vi "main 0.8.vi"() -> ()   [LabVIEW 2020]
uses:
  subvi/Newport ESP301/Newport ESP301.lvlib
  subvi/sp_manip.llb/sp_manip_lib.lvlib
  subvi/sp_manip.llb/tcp_gateway.lvlib
  subvi/PHOIBOS/DEFINITIONS/DEF_dev_type.ctl
  subvi/PHOIBOS/DEFINITIONS/DEF_dev_state.ctl
  <vilib>/Utility/file.llb/Write Delimited Spreadsheet (DBL).vi
panel:
  in  "BasePath":path=path "Z:/PESdata"
  in  "cam_liveavg":bool caption="live average"
  out "G2":dbl[](graph)
  out "cam_fps":dbl=19.67681433793903 caption="FPS" format="%.1g"
  out "sideimg":dbl[][](graph)
  out "RunNumber":u16=4
  out "sum":dbl=3886353.0 format="%#.2g"
  out "max":dbl=54.0
  out "mainimg":dbl[][](graph)
  out "ESP_con?":bool=TRUE caption="ESP301"
  out "phoib_con?":bool caption="PHOIBOS"
  out "manip_con?":bool caption="manipulator"
  out "cam_con?":bool caption="camera"
  in  "main_close":bool
  in  "Tab Control":T1(tab)
  in  "manip_deltas":dbl[](array[numeric])=[0.0, 0.0, 0.0, 0.0, 0.0, 0.0] caption="delta" format="%#.5g"
  in  "aq.mode":enum32{"Radio Selection 1", "Radio Selection 2"}(radio)
  out "snap_prog":dbl(slide) scale=0.0..1.0
  in  "upper threshold":i32=1500
  in  "dark avg":i32=20
  in  "averages":i32=20 caption="N"
  in  "ESP_delta":dbl caption="relative [mm]"
  in  "ESP_-":bool
  in  "ESP_+":bool
  in  "ESP_go":bool
  in  "ESP_dest_t":dbl caption="[fs]"
  in  "ESP_dest":dbl=33.3075 caption="[mm]"
  in  "ESP_set_t0":bool
  in  "phoib_I_6s":dbl=3200.0
  in  "phoib_I_5s":dbl=1400.0
  in  "phoib_I_4s":dbl=4.2
  in  "phoib_I_3s":dbl
  in  "phoib_I_2s":dbl=35.0
  in  "phoib_I_1s":dbl=21.9
  in  "phoib_standby":bool
  in  "phoib_set":bool
  out "phoib_I_6":dbl caption="Screen Voltage"
  out "phoib_I_5":dbl caption="Detctor Voltage"
  out "phoib_I_4":dbl caption="Work Function"
  out "phoib_I_3":dbl caption="Coil Current"
  out "phoib_I_2":dbl caption="Pass Energy"
  out "phoib_I_1":dbl caption="Kinetic Energy"
  out "Saved Positions":string[][](table)=[["ertwertwert", "-2.299945", "-2.030214", "38.900024", "50.000762", "0.000887", "-97.998082"], ["uztgugt", "-14.999451", "-13.638894", "442.380066", "13.998380", "-1.893758", "-76.305838"], ["asdf", "-14.999451", "-13.638894", "442.380066", "13.998380", "-1.893758", "-76.305838"], ["test3", "-14.999451", "-13.638894", "441.380066", "13.998380", "-1.893758", "-76.305838"]]
  in  "Save Pos":bool
  in  "Load":bool
  in  "Delete":bool
  in  "ManipRel +":bool
  in  "ManipRel -":bool
  in  "Move Abs":bool
  in  "stop manip":bool
  in  "dest":dbl[](array[numeric])=[0.007141549166819264, -0.009888298846365134, 431.30615234375, 89.00040512814502, 1.109125024699864, -227.9162918846475] caption="destination" format="%#.5g"
  out "axis":string[](array[string])=["x", "y", "z", "polar", "tilt", "azimut"]
  out "pos":dbl[](array[numeric])=[0.007141549166819264, -0.009888298846365134, 431.30615234375, 89.00040512814502, 1.109125024699864, -227.9162918846475] caption="position" format="%.5f"
  in  "Mode":T2(ring)=enum."WideAngleMode"
  in  "VoltageRange":enum16{"3.5kV", "1.5kV", "400V", "100V", "10V"}(ring)=enum."400V"
  out "ESP_pos":dbl=33.3075 caption="Position"
  out "ESP_delay":dbl caption="Delay"
  out "ESP_t0":dbl=33.3075 caption="Time Zero @"
  out "phoib_I_7":dbl caption="Conversion Voltage"
  in  "phoib_I_7s":dbl
  in  "phoib_I_8s":dbl
  in  "phoib_I_9s":dbl
  out "phoib_I_8":dbl caption="FD1"
  out "phoib_I_9":dbl caption="FD2"
  in  "gain":bool
  in  "exposure [ms]":u32=20
  in  "binning":u16(ring)=2 items=["X 1", "X 2", "X 4", "X 8"]
  in  "cam_dark?":bool caption="subtract dark?"
  in  "cam_dark":bool
  in  "cam_saveimg":bool
  in  "e-size":u8
  in  "lower threshold":i32=100
  in  "count?":bool
  out "ETA":timestamp format="%<%H:%M:%S>T"
  in  "ROI Left":i32=1
  in  "ROI Right":i32=40
  in  "ROI Top":i32=1
  in  "ROI Bottom":i32=32
  in  "delscan_iters":u32 caption="iterations"
  out "scangraph":cluster{dbl[], dbl[]}(graph)
  in  "delscan_abort":bool
  out "delscan_progress":u32(slide) scale=0.0..20.0
  in  "delscan_go":bool
  out "delscan_pos":dbl caption="current delay [fs]"
  in  "delscan_end":dbl caption="end [fs]"
  in  "delscan_stepsize":dbl caption="stepsize [fs]"
  in  "delscan_start":dbl caption="start [fs]"
  in  "comment":string
  out "iteration":i32
  out "opti_frames":dbl=25.0 caption="#steps_opti"
  out "opti_current_frame":i32=25
  out "Measurement Progress":u8(slide) scale=0.0..100.0
  out "Camera Aquisition":u8(slide) scale=0.0..100.0
  in  "Optimize":bool
  in  "OptiStepSize":dbl=-1.0 caption="Step Size"
  in  "OptiRange":dbl=25.0 caption="Range"
  in  "meas_axis":string(combo)="tilt" caption="Axis"
  in  "meas_avg":i32=60 caption="Frames2Average"
  in  "OptiCancel":bool
  out "#steps_opti":dbl=25.0
  out "current_step_opti":i32=25
  out "ETA":string
  out "manip_error":errorcluster
  out "esp_error":errorcluster
  in  "manip_init":bool
  in  "manip_release":bool
  in  "phoib_init":bool
  in  "phoib_release":bool
  in  "ESP_init":bool
  in  "ESP_release":bool
  in  "ESP301 VISA":refnum<visa-resource-name>="COM8"
  in  "board number":i32
  in  "cam_init":bool
  in  "cam_release":bool
  out "cam_error":errorcluster
  out "phoib_error":errorcluster
  out "state":T3 items=["Off"=-1, "Standby"=0, "On"=1]
  in  "ESP Axis":i32=1 min=1 max=3
  # "camera"
  # "analyzer"
  # "manipulator"
  # "aquisition"
  # "delay stage"
  # "Position"
  # "Destination"
  # "step _ of _"
  # "step _ of _"
  # "camera"
  # "phoibos"
  # "ESP301"
  # "manipulator"
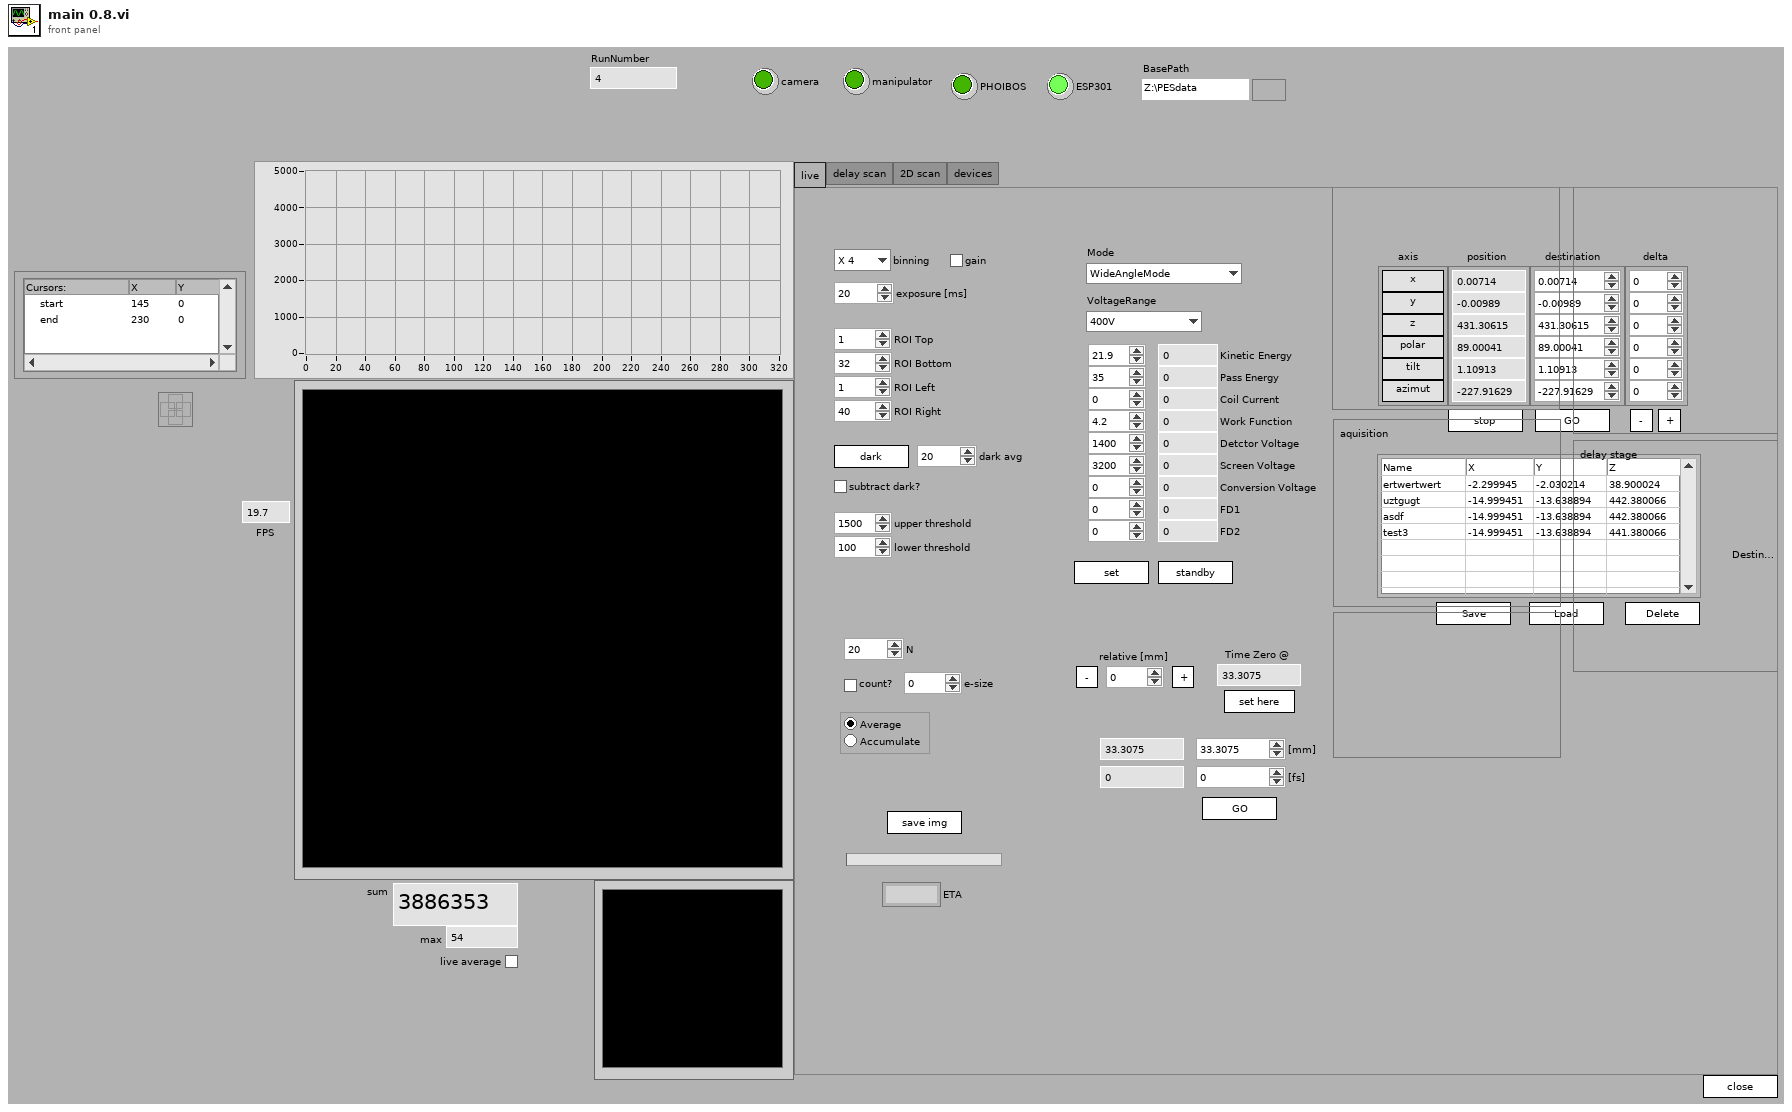
[diagram p1: front panel]
types:
  T1 = enum32{"live", "delay scan", "2D scan", "devices"}
  T2 = enum16{"HighMagnification", "MediumMagnification", "LowMagnification", "HighAngularDispersion", "MediumAngularDispersion", "LowAngularDispersion", "WideAngleMode", "LargeArea", "MediumArea", "SmallArea", "HighMagnification2", "SmallArea2", "ImagingMode"}
  T3 = typedef "DEF_dev_state.ctl" = i32
  T4 = typedef "LVCursorListTypeDef.ctl" = cluster{"Name":string, "Color":u32, "Style":u8, "Point Style":u8, "Name Visible":bool, "Allow Drag":bool, "Cursor Mode":u32, "Plot":i32, "Index":i32, "Position":cluster{"X":dbl, "Y":dbl}, "X Scale":u32, "Y Scale":u32, "Watch Plots":i32[], "Watch All Plots":bool, "Plot Area":i32, "Label Offset":cluster{"X":dbl, "Y":dbl}}[]
  T5 = cluster{"Name":string, "Color":u32, "Style":u8, "Point Style":u8, "Name Visible":bool, "Allow Drag":bool, "Cursor Mode":u32, "Plot":i32, "Index":i32, "Position":cluster{"X":dbl, "Y":dbl}, "X Scale":u32, "Y Scale":u32, "Watch Plots":i32[], "Watch All Plots":bool, "Plot Area":i32, "Label Offset":cluster{"X":dbl, "Y":dbl}}
  T6 = cluster{"Camera type":u32, "Operating mode\nHP & QE / HS & DiCam Pro ":u32, "Frame trigger \n(High Performance and QE only)":u16, "Sequence trigger":u16, "Low Light\n(QE only)":bool, "Gain":bool, "Horzontal\nbinning":u16, "Vertical\nbinning ":u16, "ROI Left":i32, "ROI Right":i32, "ROI Top":i32, "ROI Bottom":i32}
  T7 = cluster{"Axis_Name":string, "Axis_Type":string, "Axis_Position":dbl, "continous":bool, "moving":bool}[]
  T8 = typedef "DEF_dev_type.ctl" = enum32{"devA (analyzer)", "devD (detector)"}
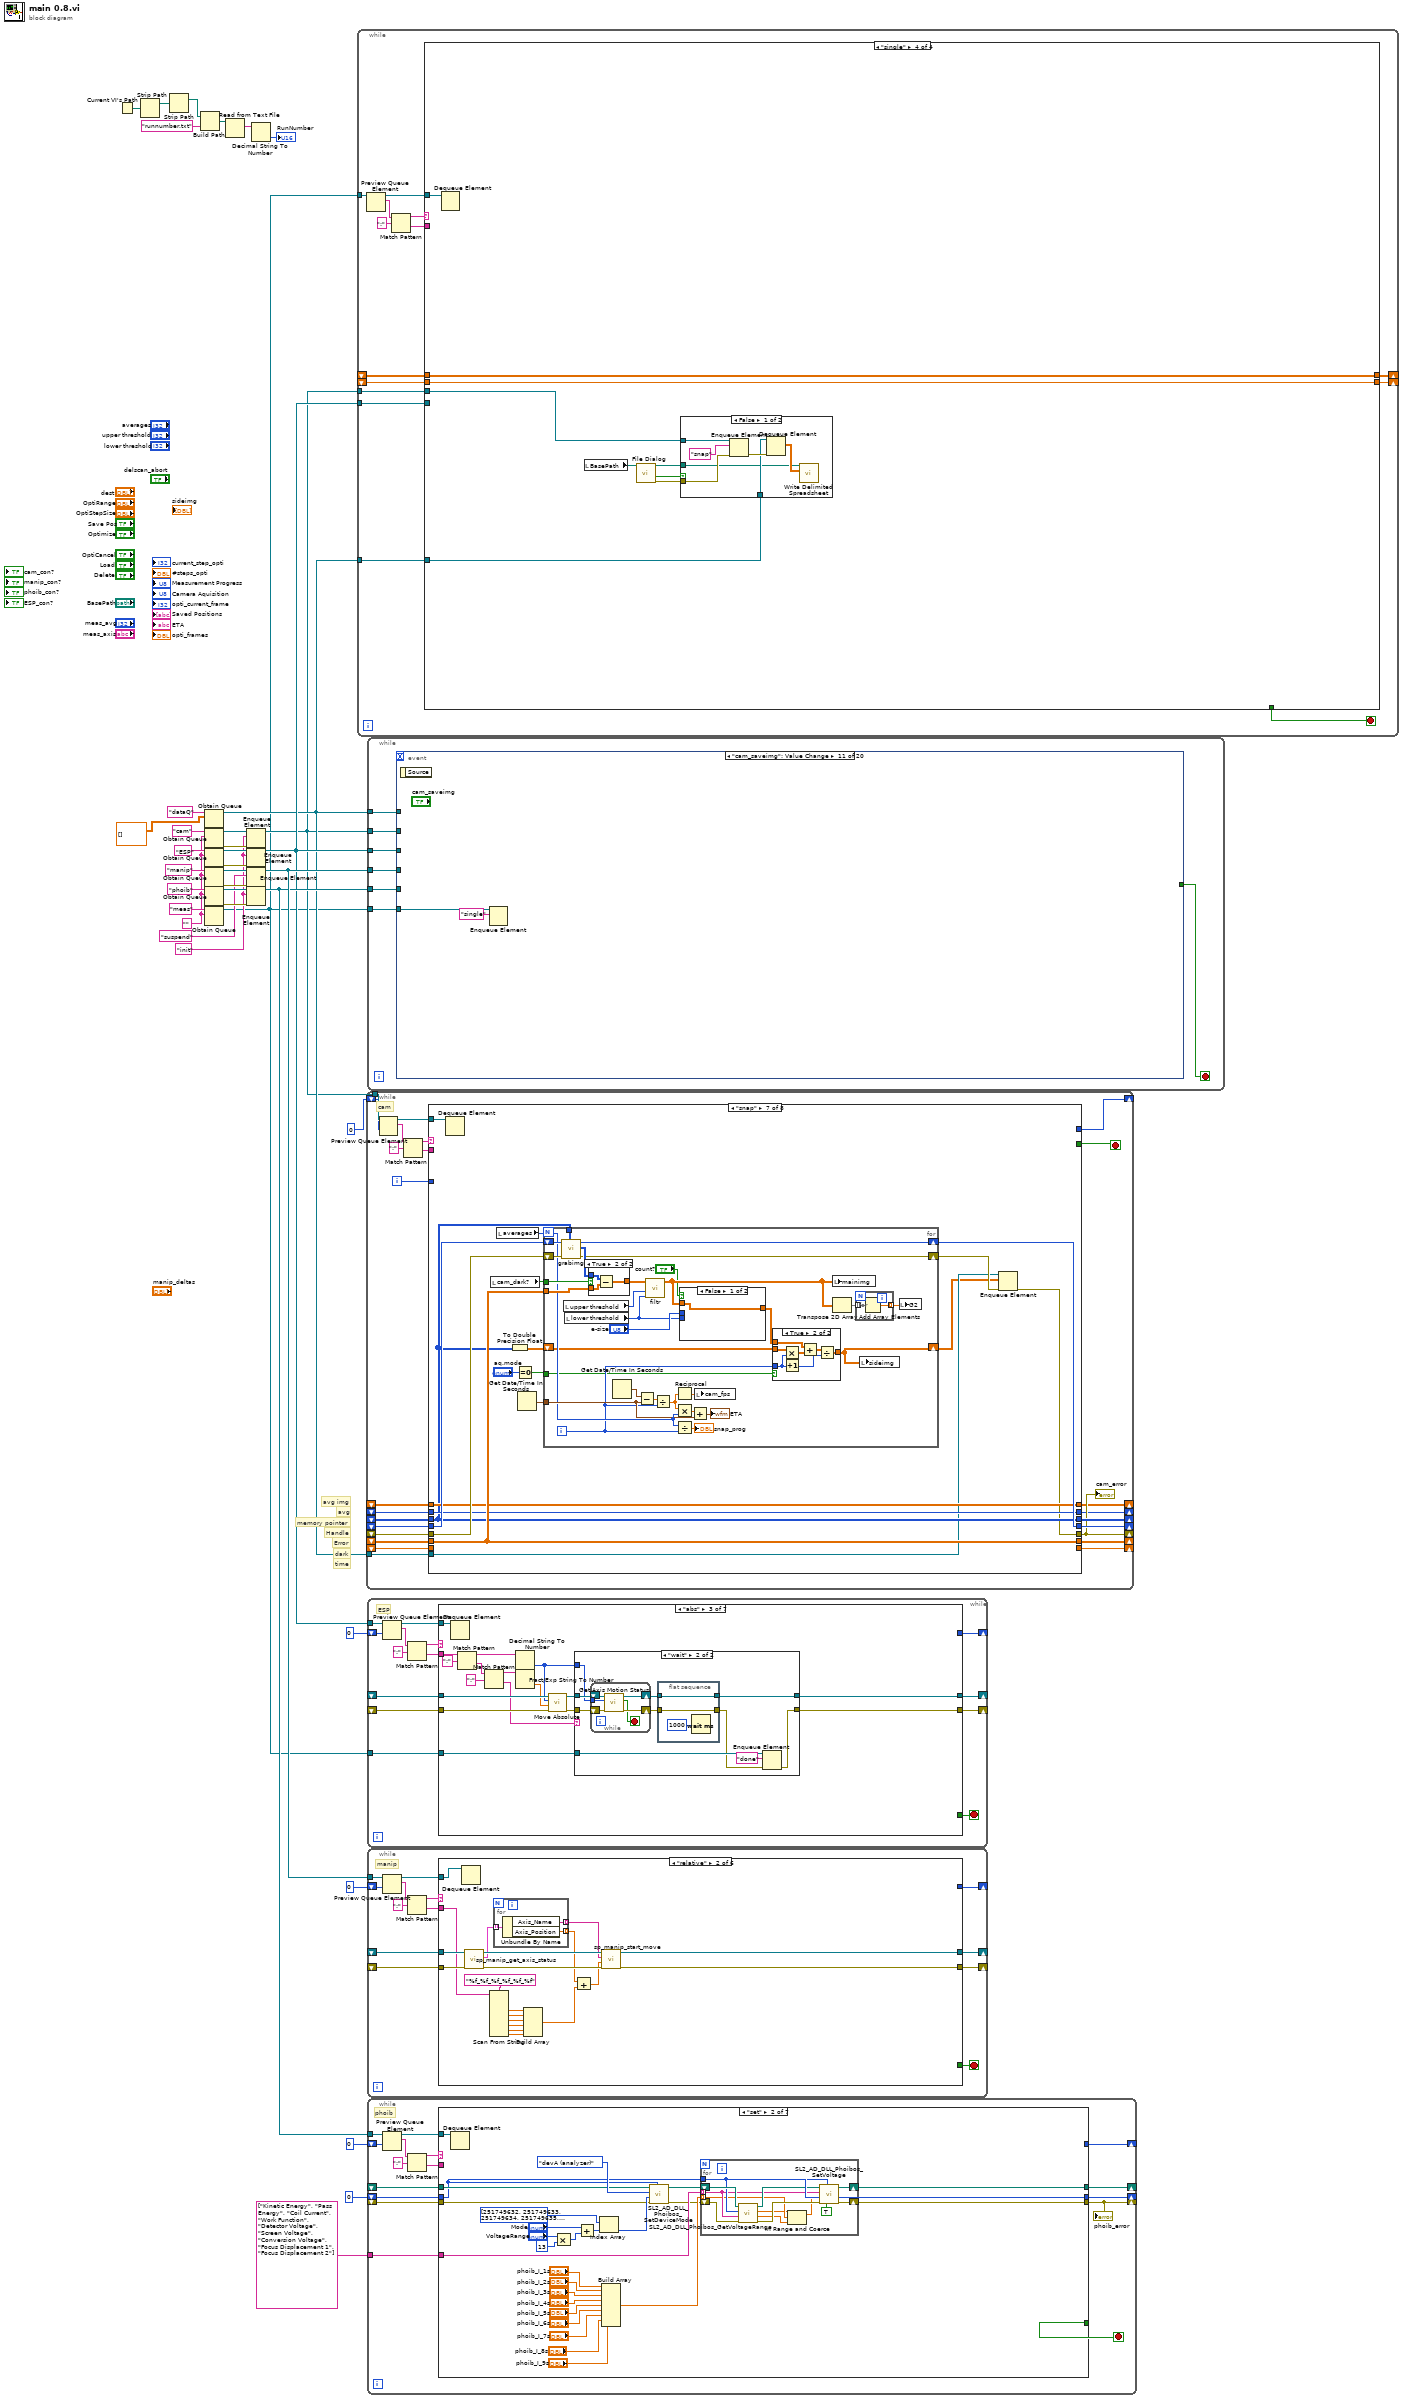
[diagram p0: block diagram]
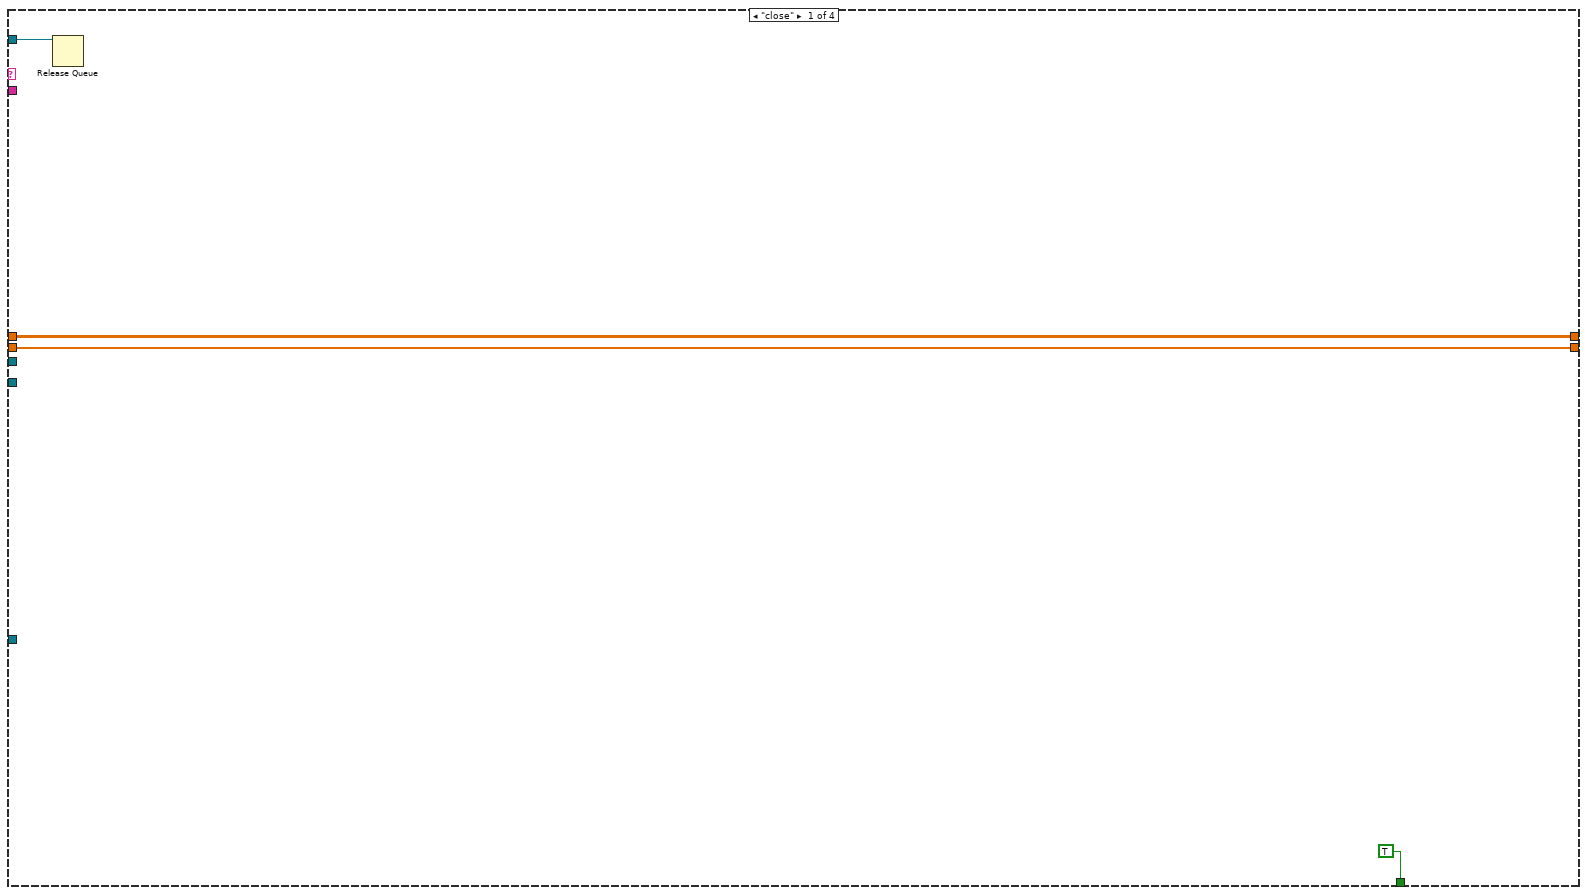
[diagram p2: hidden frame]
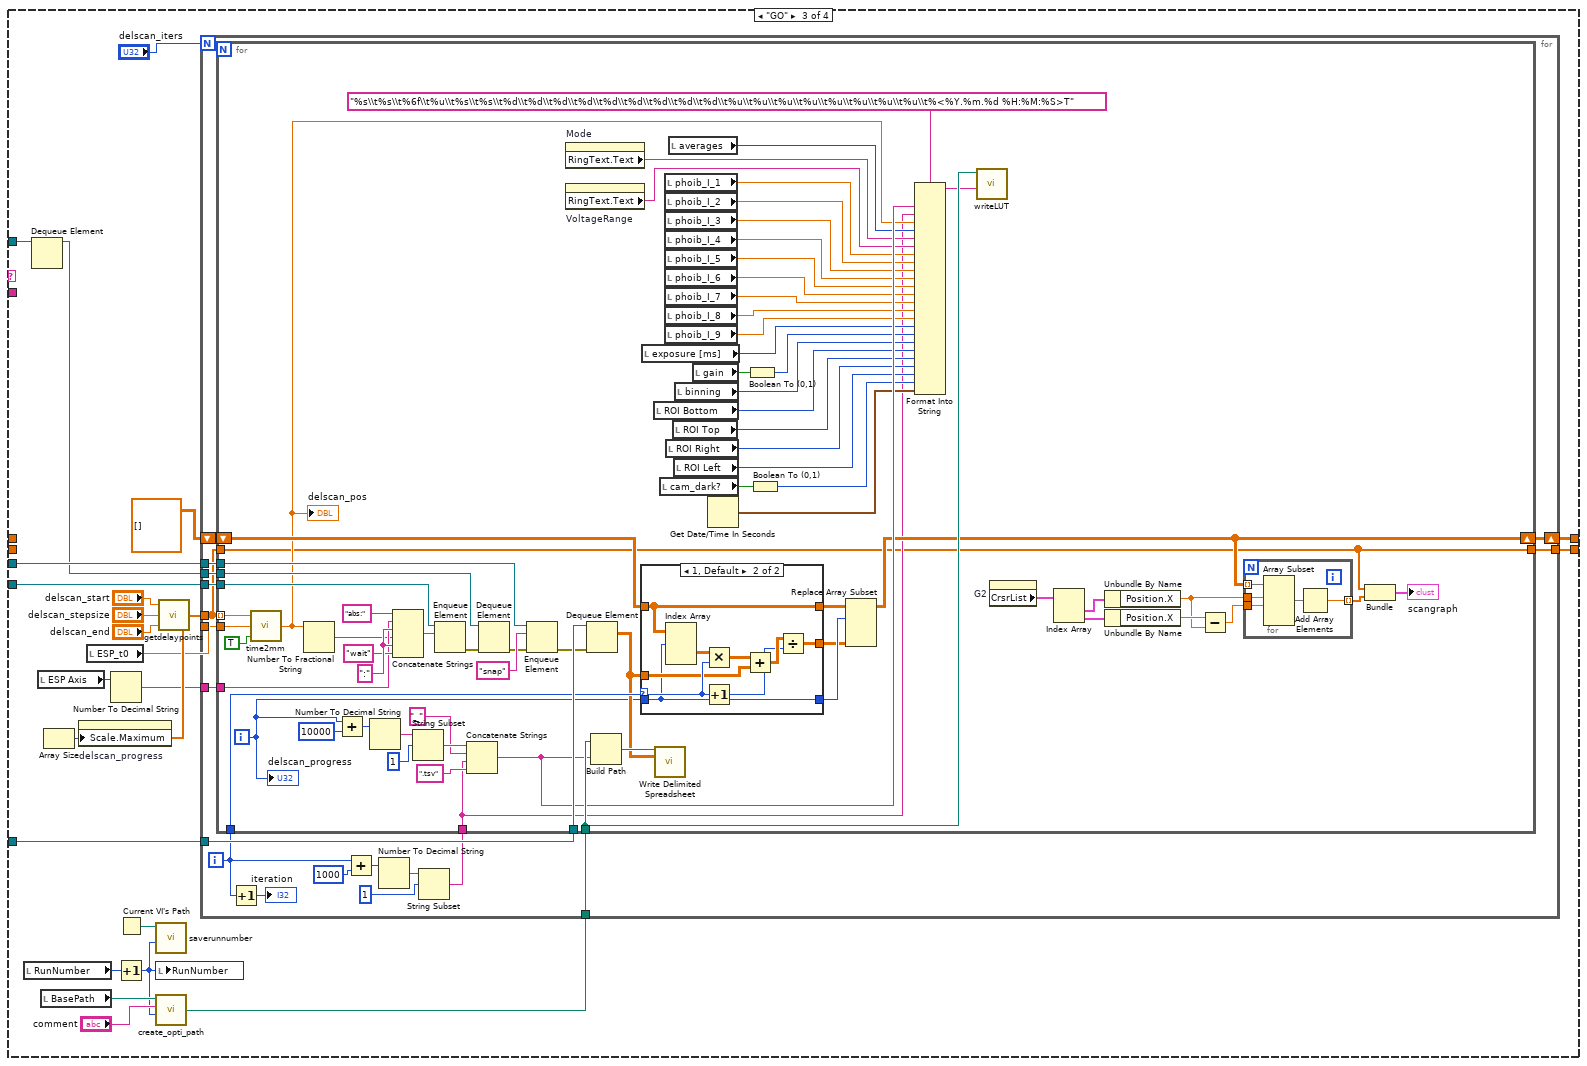
[diagram p4: hidden frame]
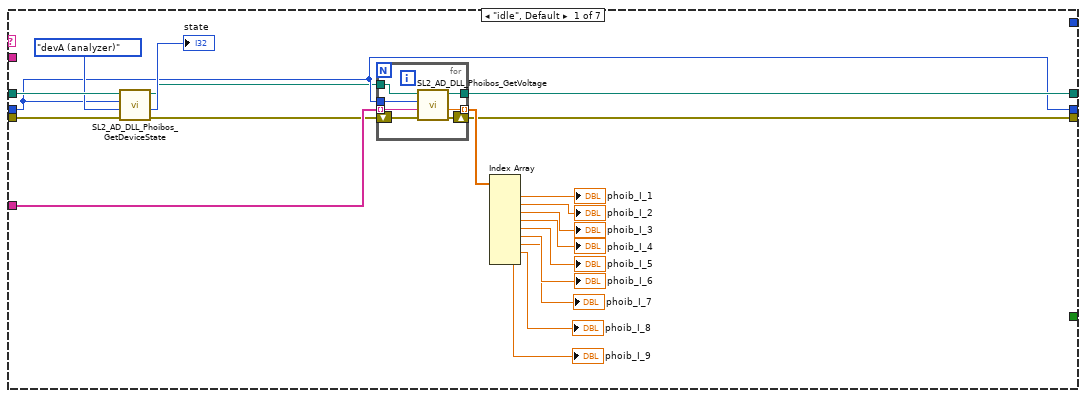
[diagram p7: hidden frame]
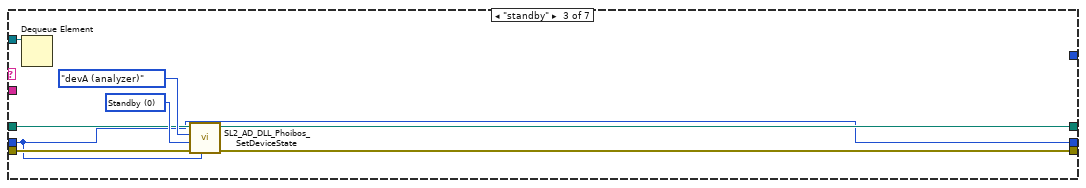
[diagram p8: hidden frame]
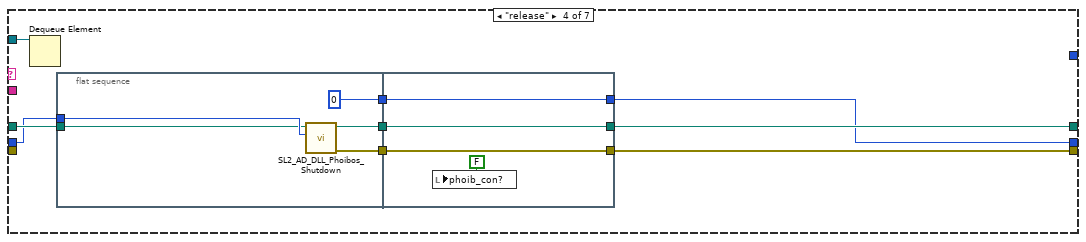
[diagram p9: hidden frame]
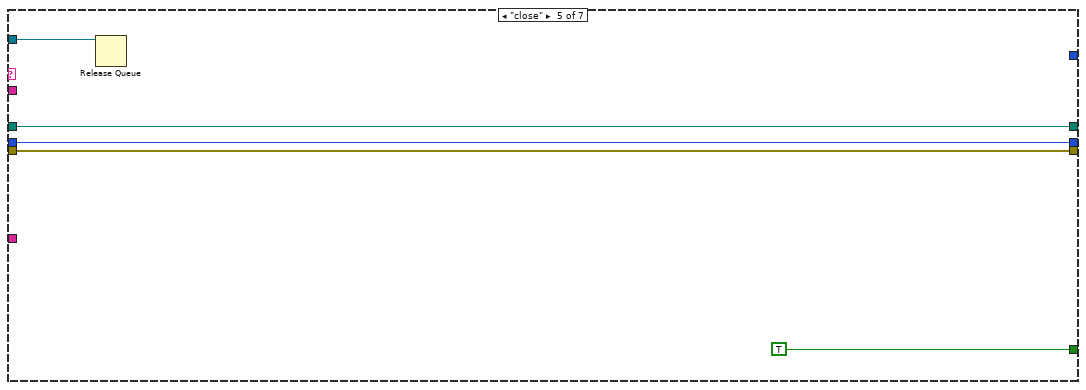
[diagram p10: hidden frame]
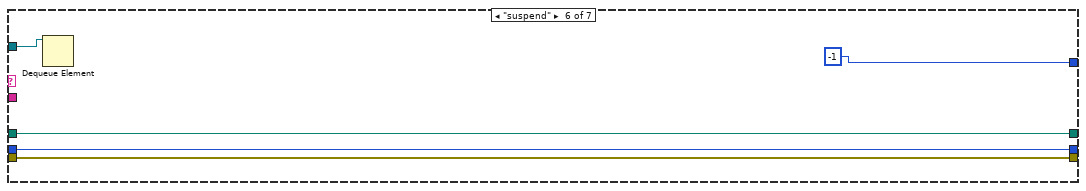
[diagram p11: hidden frame]
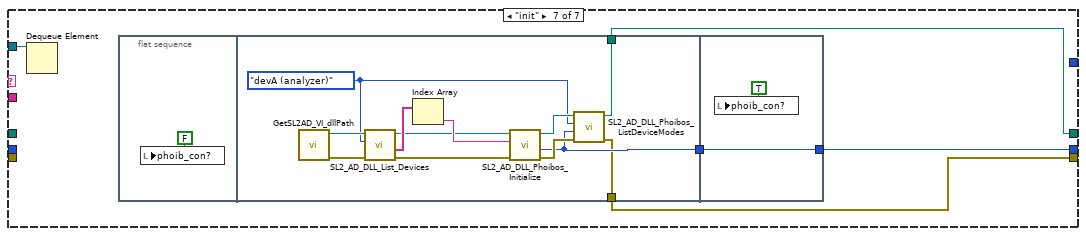
[diagram p12: hidden frame]
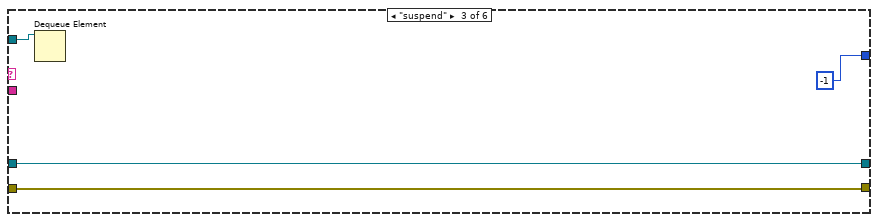
[diagram p14: hidden frame]
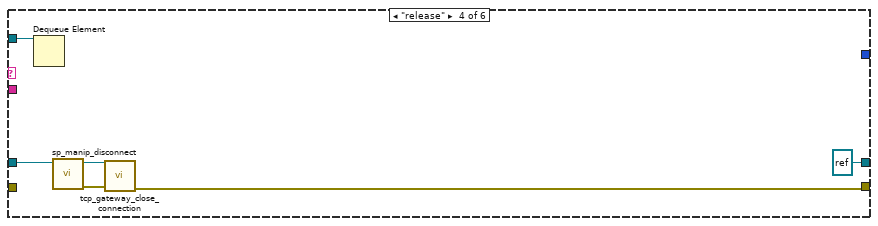
[diagram p15: hidden frame]
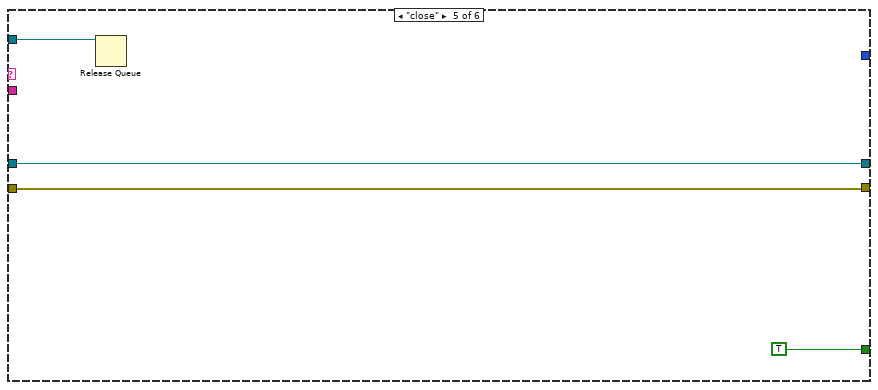
[diagram p16: hidden frame]
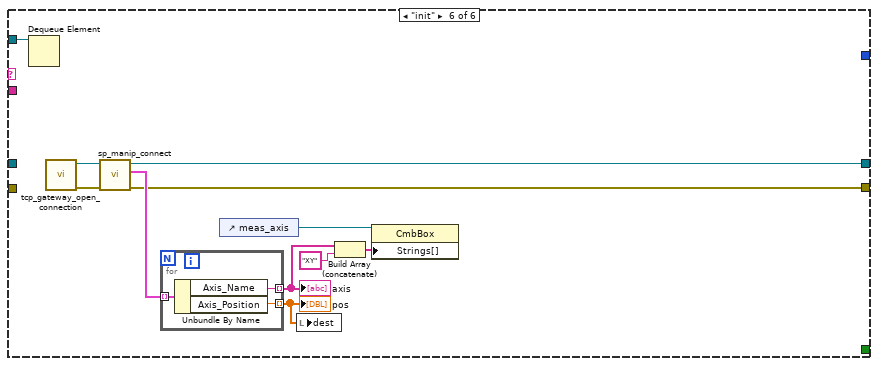
[diagram p17: hidden frame]
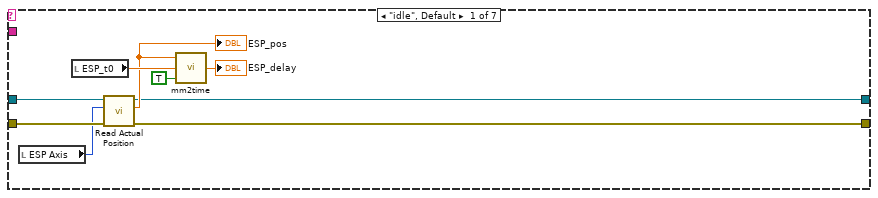
[diagram p18: hidden frame]
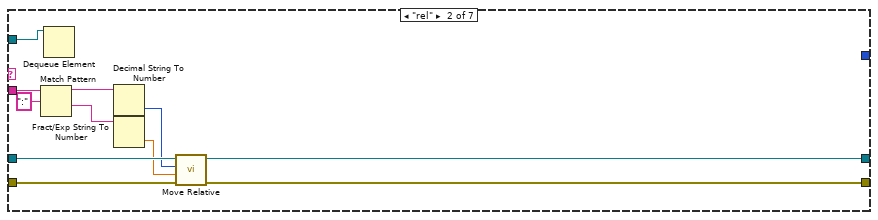
[diagram p19: hidden frame]
diagram:
  w13 = "init" ("name (unnamed)")
  w15 = "" ("name (unnamed)")
  # "avg img"
  # "avg"
  # "time"
  # "dark"
  # "Error"
  # "Handle"
  # "memory pointer"
  n1 = Current VI's Path() -> (path=w2:path)
  n2 = Strip Path(path=w2) -> (stripped path=w7:path)  [unwired: 1 out]
  n3 = Strip Path(path=w7) -> (stripped path=w8:path)  [unwired: 1 out]
  n4 = Build Path(base path=w8, name or relative path="runnumber.txt") -> (appended path=w4:path)
  n5 = Obtain Queue(name (unnamed)="dataQ", element data type=dbl[][] []) -> (queue out=w10:refnum<queue>)  [unwired: 3 in, 2 out]
  n6 = Obtain Queue(name (unnamed)="cam", element data type=w15) -> (queue out=w36:refnum<queue>, error out=w35:errorcluster)  [unwired: 3 in, 1 out]
  n7 = Obtain Queue(name (unnamed)="ESP", element data type=w15) -> (queue out=w33:refnum<queue>, error out=w34:errorcluster)  [unwired: 3 in, 1 out]
  n8 = Obtain Queue(name (unnamed)="manip", element data type=w15) -> (queue out=w30:refnum<queue>, error out=w29:errorcluster)  [unwired: 3 in, 1 out]
  n9 = Obtain Queue(name (unnamed)="phoib", element data type=w15) -> (queue out=w27:refnum<queue>, error out=w28:errorcluster)  [unwired: 3 in, 1 out]
  n10 = Obtain Queue(name (unnamed)="meas", element data type=w15) -> (queue out=w1:refnum<queue>)  [unwired: 3 in, 2 out]
  n11 = Read from Text File(file (use dialog)=w4) -> (text=w5:string)  [unwired: 3 in, 3 out]
  n12 = Enqueue Element(queue=w36, element=w13, error in (no error)=w35) -> (queue out=w9:refnum<queue>)  [unwired: 1 in, 2 out]
  n13 = Enqueue Element(queue=w33, element=w13, error in (no error)=w34) -> (queue out=w12:refnum<queue>)  [unwired: 1 in, 2 out]
  n14 = Enqueue Element(queue=w30, element="suspend" ("name (unnamed)"), error in (no error)=w29) -> (queue out=w24:refnum<queue>)  [unwired: 1 in, 2 out]
  n15 = Enqueue Element(queue=w27, element=w13, error in (no error)=w28) -> (queue out=w23:refnum<queue>)  [unwired: 1 in, 2 out]
  n16 = Decimal String To Number(string=w5) -> (number=→"RunNumber":i32)  [unwired: 2 in, 1 out]
  n17 = while {
    tunnel: w10 -> [w51]
    tunnel: w12 -> [w50]
    tunnel: w9 -> [w49]
    shift-right: [w46] -> _
    shift-left: _ -> [w48]
    shift-right: [w45] -> _
    shift-left: _ -> [w47]
    tunnel: w1 -> [w42]
    stop <- w38 stop-if-true
    n18 = Preview Queue Element(queue=w42) -> (queue out=w39:refnum<queue>, element=w44:string)  [unwired: 2 in, 2 out]
    n19 = Match Pattern(string=w44, regular expression=":") -> (before substring=w41:string, after substring=w40:string)  [unwired: 1 in, 2 out]
    n20 = case shown="\"single\"" w41 {
      tunnel: w51 -> [_ _ w80 w189]
      tunnel: w50 -> [_ _ w79 _]
      tunnel: w49 -> [_ _ w78 w191]
      tunnel: w48 -> [w53 w57 _ w188]
      tunnel: w47 -> [w52 w56 _ w187]
      tunnel: [w53 w57 w77 w188] -> w46
      tunnel: [w52 w56 w58 w187] -> w45
      tunnel: w40 -> [_ _ _ _]
      tunnel: w39 -> [w55 _ w60 w190]
      tunnel: [TRUE _ _ _] -> w38
      frame "close" {
        n21 = Release Queue(queue=w55) -> ()  [unwired: 2 in, 3 out]
      }
      frame "idle", Default {
      }
      frame "GO" {
        n22 = local read "RunNumber"() -> (w75:u16)
        n23 = Dequeue Element(queue=w60) -> (queue out=w59:refnum<queue>)  [unwired: 2 in, 3 out]
        n24 = local read "ESP Axis"() -> (w71:i32)
        n25 = local read "BasePath"() -> (w73:path)
        n26 = local read "ESP_t0"() -> (w64:dbl)
        n27 = Number To Decimal String(number=w71) -> (decimal integer string=w63:string)  [unwired: 1 in]
        n28 = Increment(x=w75) -> (x+1=w72:u16)
        n29 = Current VI's Path() -> (path=w76:path)
        n30 = call "saverunnumber.vi"("RunNumber"=w72, "VI path"=w76) -> ()  [unwired: 10 in]
        n31 = local write "RunNumber"(w72) -> ()
        n32 = call "create_opti_path.vi"("RunNumber"=w72, 3:"comment", "base path"=w73) -> ("Path"=w62:path)  [unwired: 1 in]
        n33 = call "getdelaypoints.vi"("delscan_stepsize"="delscan_end", "delscan_end"="delscan_stepsize", "delscan_start"="delscan_start") -> ("delaypoints"=w65:dbl[])
        n34 = Array Size(array=w65) -> (size(s)=w67:i32)
        n35 = property on="delscan_progress" class="Slide (strict)"("Scale.Maximum"=w67) -> ()  [unwired: 2 in, 2 out]
        n36 = for {
          N: "delscan_iters" -> [_]
          tunnel: w65 -> [w82]
          tunnel: w64 -> [w98]
          tunnel: w63 -> [w97]
          tunnel: w79 -> [w95]
          tunnel: w80 -> [w94]
          tunnel: w59 -> [w93]
          tunnel: w78 -> [w92]
          tunnel: w62 -> [w91]
          shift-right: [w89] -> w77
          shift-left: dbl[][][] [] -> [w90]
          tunnel: [w81] -> w58
          i -> [w84]
          n37 = Increment(x=w84) -> (x+1=→"iteration":i32)
          n38 = Add(x=w84, y=1000) -> (x+y=w87:i32)
          n39 = Number To Decimal String(number=w87) -> (decimal integer string=w86:string)  [unwired: 1 in]
          n40 = String Subset(string=w86, offset (0)=1) -> (substring=w83:string)  [unwired: 1 in]
          n41 = for {
            tunnel: w82 -> [w163] mode=indexing
            tunnel: w98 -> [w142]
            tunnel: w97 -> [w162]
            tunnel: w95 -> [w161]
            tunnel: w94 -> [w149]
            tunnel: w93 -> [w160]
            tunnel: w92 -> [w159]
            tunnel: w91 -> [w146]
            shift-right: [w106] -> w89
            shift-left: w90 -> [w128]
            tunnel: w84 -> [w127]
            tunnel: w83 -> [w100]
            tunnel: w82 -> [w99]
            tunnel: [w99] -> w81
            i -> [w122]
            w165 = ":" ("string")
            n42 = call "time2mm.vi"("fs[1]/ps[0]"=TRUE, "Offset (mm)"=w142, "time"=w163) -> ("position (mm)"=w121:dbl)
            "delscan_pos" <- w121
            n43 = Number To Fractional String(number=w121) -> (F-format string=w143:string)  [unwired: 3 in]
            n44 = Add(x=w122, y=10000) -> (x+y=w157:i32)
            n45 = Number To Decimal String(number=w157) -> (decimal integer string=w156:string)  [unwired: 1 in]
            n46 = Concatenate Strings("abs:" ("string"), w162, w165, w143, w165, "wait" ("string")) -> (w169:string)
            n47 = String Subset(string=w156, offset (0)=1) -> (substring=w154:string)  [unwired: 1 in]
            n48 = Enqueue Element(queue=w161, element=w169) -> (error out=w166:errorcluster)  [unwired: 2 in, 2 out]
            n49 = Concatenate Strings(w154, "_" ("string"), w100, ".tsv" ("string")) -> (w144:string)
            n50 = Dequeue Element(queue=w160, error in (no error)=w166) -> (error out=w150:errorcluster)  [unwired: 1 in, 3 out]
            n51 = Enqueue Element(queue=w159, element="snap", error in (no error)=w150) -> (error out=w148:errorcluster)  [unwired: 1 in, 2 out]
            n52 = property on="Mode" class="Enum (strict)"() -> ("RingText.Text"=w140:string)  [unwired: 2 in, 2 out]
            n53 = property on="VoltageRange" class="Enum (strict)"() -> ("RingText.Text"=w139:string)  [unwired: 2 in, 2 out]
            n54 = Dequeue Element(queue=w149, error in (no error)=w148) -> (element=w126:dbl[][])  [unwired: 1 in, 3 out]
            n55 = Build Path(base path=w146, name or relative path=w144) -> (appended path=w147:path)
            n56 = case shown="1, Default" w127 {
              selector: w127 -> [w175 w185]
              tunnel: w128 -> [w177 w178]
              tunnel: w122 -> [_ w179]
              tunnel: w126 -> [w176 w181]
              tunnel: [w177 w178] -> w125
              tunnel: [w176 w182] -> w123
              tunnel: [w175 w179] -> w124
              frame 0 {
              }
              frame 1, Default {
                n57 = Index Array(array=w178, index (dim 0)=w179) -> (element=w186:dbl[][])  [unwired: 2 in]
                n58 = Multiply(x=w186, y=w185) -> (x*y=w180:dbl[][])
                n59 = Increment(x=w185) -> (x+1=w183:i32)
                n60 = Add(x=w180, y=w181) -> (x+y=w184:dbl[][])
                n61 = Divide(x=w184, y=w183) -> (x/y=w182:dbl[][])
              }
            }
            n62 = local read "exposure [ms]"() -> (w120:u32)
            n63 = local read "ROI Bottom"() -> (w118:i32)
            n64 = call-poly <vilib>:"Write Delimited Spreadsheet.vi"("file path (dialog if empty)"=w147, "2D data"=w126) -> ()  [unwired: 12 in, 2 out]
            n65 = local read "cam_dark?"() -> (w111:bool)
            n66 = local read "phoib_I_1"() -> (w138:dbl)
            n67 = local read "phoib_I_2"() -> (w137:dbl)
            n68 = local read "phoib_I_3"() -> (w136:dbl)
            n69 = local read "phoib_I_4"() -> (w135:dbl)
            n70 = local read "phoib_I_5"() -> (w134:dbl)
            n71 = local read "phoib_I_6"() -> (w133:dbl)
            n72 = local read "phoib_I_7"() -> (w132:dbl)
            n73 = local read "phoib_I_8"() -> (w131:dbl)
            n74 = local read "phoib_I_9"() -> (w130:dbl)
            n75 = local read "ROI Right"() -> (w116:i32)
            n76 = local read "averages"() -> (w141:i32)
            n77 = local read "ROI Top"() -> (w117:i32)
            n78 = local read "ROI Left"() -> (w115:i32)
            n79 = local read "binning"() -> (w119:u16)
            n80 = local read "gain"() -> (w113:bool)
            n81 = Get Date/Time In Seconds() -> (seconds since 1Jan1904=w114:timestamp)
            n82 = Boolean To (0,1)(Boolean=w113) -> (0, 1=w112:i16)
            n83 = Boolean To (0,1)(Boolean=w111) -> (0, 1=w110:i16)
            n84 = Replace Array Subset(array=w125, new element=w123, index (dim 0)=w124) -> (w106:dbl[][][])  [unwired: 2 in]
            n85 = Format Into String(format string="%s\\t%s\\t%6f\\t%u\\t%s\\t%s\\t%d\\t%d\\t%d\\t%d\\t%d\\t%d\\t%d\\t%d\\t%d\\t%u\\t%u\\t%u\\t%u\\t%u\\t%u\\t%u\\t%u\\t%<%Y.%m.%d %H:%M:%S>T", w144, w100, w121, w141, w140, w139, w138, w137, w136, w135, w134, w133, w132, w131, w130, w120, w112, w119, w118, w117, w116, w115, w110, w114) -> (resulting string=w129:string)  [unwired: 2 in, 1 out]
            n86 = call "writeLUT.vi"("text"=w129, "base path"=w146) -> ()  [unwired: 10 in]
            n87 = property on="G2" class="WFGraph (strict)"() -> ("CrsrList"=w109:T4)  [unwired: 2 in, 2 out]
            n88 = Index Array(array=w109) -> (element #1=w108:T5, element #2=w107:T5)  [unwired: 2 in]
            n89 = Unbundle By Name(w108) -> ("Position.X"=w104:dbl)
            n90 = Unbundle By Name(w107) -> ("Position.X"=w105:dbl)
            n91 = Subtract(x=w105, y=w104) -> (x-y=w103:dbl)
            n92 = for {
              tunnel: w106 -> [w174] mode=indexing
              tunnel: w104 -> [w173]
              tunnel: w103 -> [w172]
              tunnel: [w170] -> w102 mode=indexing
              n93 = Array Subset(array=w174, index (row)=w173, length (row)=w172) -> (w171:dbl[][])  [unwired: 2 in]
              n94 = Add Array Elements(numeric array=w171) -> (sum=w170:dbl)
            }
            n95 = Bundle("delaypoints"=w99, w102) -> (→"scangraph":cluster{"delaypoints":dbl[], dbl[]})  [unwired: 1 in]
            "delscan_progress" <- w122
          }
        }
      }
      frame "single" {
        n96 = Dequeue Element(queue=w190) -> ()  [unwired: 2 in, 4 out]
        n97 = local read "BasePath"() -> (w195:path)
        n98 = call "File Dialog"("start path"=w195) -> ("selected path"=w193:path, "cancelled"=w194:bool, "error out"=w192:errorcluster)  [unwired: 11 in, 1 out]
        n99 = case shown="False" w194 {
          tunnel: w193 -> [w196 _]
          tunnel: w192 -> [w201 _]
          tunnel: w191 -> [w202 _]
          tunnel: w189 -> [w198 _]
          frame False {
            n100 = Enqueue Element(queue=w202, element="snap" ("string"), error in (no error)=w201) -> (error out=w199:errorcluster)  [unwired: 1 in, 2 out]
            n101 = Dequeue Element(queue=w198, error in (no error)=w199) -> (element=w197:dbl[][])  [unwired: 1 in, 3 out]
            n102 = call-poly <vilib>:"Write Delimited Spreadsheet.vi"("file path (dialog if empty)"=w196, "2D data"=w197) -> ()  [unwired: 12 in, 2 out]
          }
          frame True {
          }
        }
      }
    }
  }
  n103 = while {
    tunnel: w9 -> [w227]
    shift-right: [w221] -> _
    shift-left: _ -> [w220]
    shift-right: [w219] -> _
    shift-left: _ -> [w217]
    shift-right: [w218] -> _
    shift-left: _ -> [w216]
    shift-right: [w213] -> _
    shift-left: 0 -> [w214]
    shift-right: [w212] -> _
    shift-left: _ -> [w211]
    shift-right: [w210] -> _
    shift-left: _ -> [w209]
    tunnel: w10 -> [w208]
    shift-right: [w207] -> _
    shift-left: _ -> [w206]
    shift-right: [w204] -> _
    shift-left: _ -> [w203]
    i -> [w205]
    stop <- w215 stop-if-true
    # "cam"
    n104 = Preview Queue Element(queue=w227, timeout in ms (-1)=w214) -> (queue out=w226:refnum<queue>, element=w225:string)  [unwired: 1 in, 2 out]
    n105 = Match Pattern(string=w225, regular expression=":") -> (before substring=w222:string, after substring=w223:string)  [unwired: 1 in, 2 out]
    n106 = case shown="\"snap\"" w222 {
      tunnel: w226 -> [w237 w267 w295 w307 _ w364 w392 w455]
      tunnel: w223 -> [_ _ _ _ _ _ _ _]
      tunnel: [w231 w253 w294 w305 w312 w361 w381 w453] -> w221
      tunnel: w220 -> [_ _ w294 w305 w312 w361 w381 w453]
      tunnel: [w236 w268 u64 0 ("Hout") w304 w322 w362 w387 w452] -> w219
      tunnel: [w238 w269 w291 w303 w323 w363 w375 w451] -> w218
      tunnel: w217 -> [_ w271 w293 w304 w325 w366 w389 w452]
      tunnel: w216 -> [_ w270 _ w303 w324 w365 w388 w451]
      tunnel: [_ _ _ TRUE _ _ _ _] -> w215
      tunnel: [_ _ _ _ _ _ _ -1] -> w213
      tunnel: [w230 w254 _ _ w333 _ _ _] -> w212
      tunnel: w211 -> [w230 w254 _ _ w332 _ _ _]
      tunnel: [w231 w256 w289 w302 w328 w355 w390 w450] -> w210
      tunnel: w209 -> [_ w256 w289 w302 w328 _ w390 w450]
      tunnel: w208 -> [_ _ _ _ _ _ w379 _]
      tunnel: [w228 w251 w288 w300 w309 w352 w384 w449] -> w207
      tunnel: w206 -> [w228 w251 w288 w300 w316 w352 w384 w449]
      tunnel: w205 -> [_ _ _ _ w315 _ _ _]
      tunnel: [w229 w252 w287 w301 w314 w351 w383 w448] -> w204
      tunnel: w203 -> [w229 w252 w287 w301 w313 w351 w383 w448]
      frame "init" {
        w231 = u16[][] []
        n107 = flat-sequence {
          tunnel: [w240] -> w235
          tunnel: [w241] -> w234
          tunnel: [w249] -> w236
          tunnel: [w250] -> w238
          tunnel: w235 -> [w250]
          tunnel: w234 -> [w249]
          frame #0 {
            n108 = local write "cam_con?"(FALSE ("cam_con?")) -> ()
          }
          frame #1 {
            n109 = call "SCInitBoard.vi"("boardnr"="board number") -> ("Hout"=w244:u32, "error out"=w245:errorcluster)  [unwired: 1 in, 1 out]
            n110 = call "SCSetupCamera.vi"("Handle"=w244, "error in (no error)"=w245) -> ("Hout"=w246:u64, "error out"=w247:errorcluster)  [unwired: 1 out]
            n111 = call "SCStopCOC.vi"("error in (no error)"=w247, "Stop mode"=0, "Handle"=w246) -> ("error out"=w240:errorcluster, "Hout"=w241:u64)
          }
          frame #2 {
            n112 = local write "cam_con?"(TRUE ("cam_con?")) -> ()
          }
        }
        n113 = Dequeue Element(queue=w237) -> (queue out=w233:refnum<queue>)  [unwired: 2 in, 3 out]
        n114 = Enqueue Element At Opposite End(queue=w233, element="set") -> ()  [unwired: 2 in, 3 out]
      }
      frame "set" {
        w266 = u32 1 ("Operating mode\nHP & QE / HS & DiCam Pro")
        n115 = Dequeue Element(queue=w267) -> ()  [unwired: 2 in, 4 out]
        n116 = Bundle By Name(cluster=cluster{"Delay":dbl, "Exposure ":dbl} {"Delay"=0.0, "Exposure "=0.0} ("Delay and exposure"), "Exposure"="exposure [ms]") -> (w263:cluster{"Delay":dbl, "Exposure ":dbl})
        n117 = call "SCStopCOC.vi"("error in (no error)"=w270, "Stop mode"=0, "Handle"=w271) -> ("error out"=w286:errorcluster, "Hout"=w285:u64)
        n118 = Bundle By Name(cluster=T6 {"Camera type"=0, "Operating mode\nHP & QE / HS & DiCam Pro "=0, "Frame trigger \n(High Performance and QE only)"=0, "Sequence trigger"=0, "Low Light\n(QE only)"=FALSE, "Gain"=FALSE, "Horzontal\nbinning"=0, "Vertical\nbinning "=0, "ROI Left"=1, "ROI Right"=20, "ROI Top"=1, "ROI Bottom"=15} ("Camera controls"), "Operating mode\nHP & QE / HS & DiCam Pro"=w266, "Horzontal\nbinning"="binning", "Vertical\nbinning"="binning", "ROI Left"="ROI Left", "ROI Right"="ROI Right", "ROI Top"="ROI Top", "ROI Bottom"="ROI Bottom", "Gain"="gain") -> (w281:T6)
        n119 = call "New delay and exposure forma.vi"("Operating mode\nHP & QE / HS & DiCam Pro"=w266, "Delay and exposure"=w263) -> ("Output table"=w282:string)  [unwired: 3 in]
        n120 = call "SCSetCoC.vi"("error in (no error)"=w286, "Delay and exposure table"=w282, "Camera controls"=w281, "Handle"=w285) -> ("error out"=w274:errorcluster, "Hout"=w273:u64)  [unwired: 1 out]
        n121 = call "SCGetImageSize.vi"("Handle"=w273, "error in (no error)"=w274) -> ("Hout"=w272:u64, "error out"=w255:errorcluster, "Horizontal size"=w260:i32, "Vertical size"=w259:i32)  [unwired: 2 out]
        n122 = Greater?(x=w260, y=w259) -> (0:w261:bool)
        n123 = Initialize Array(u16 0 ("dimension size"), w259, w260) -> (w253:u16[][])
        n124 = call "SCRun.vi"("error in (no error)"=w255, "Run mode"=0, "Handle"=w272) -> ("error out"=w269:errorcluster, "Hout"=w268:u64)  [unwired: 1 out]
        n125 = Select(t=w260, s=w261, f=w259) -> (s? t:f=w258:i32)
        n126 = property on="mainimg" class="IntGraph (strict)"("XScale.Maximum"=w258, "YScale.Maximum"=w258) -> ()  [unwired: 2 in, 2 out]
      }
      frame "release" {
        n127 = Dequeue Element(queue=w295) -> ()  [unwired: 2 in, 4 out]
        n128 = flat-sequence {
          tunnel: w293 -> [w297]
          tunnel: [w296] -> w290
          tunnel: [w299] -> w291
          tunnel: w290 -> [w299]
          frame #0 {
            n129 = call "SCCloseBoard.vi"("Handle"=w297) -> ("error out"=w296:errorcluster)  [unwired: 1 in, 2 out]
          }
          frame #1 {
            n130 = local write "cam_con?"(FALSE ("cam_con?")) -> ()
          }
        }
      }
      frame "close" {
        n131 = Release Queue(queue=w307) -> ()  [unwired: 2 in, 3 out]
      }
      frame "idle", Default {
        n132 = call "grabimg.vi"("array in"=w312, "error in"=w324, "Hin"=w325) -> ("error out"=w323:errorcluster, "imgdata"=w321:i32[][], "Hout"=w322:u64)  [unwired: 6 in]
        n133 = local read "upper threshold"() -> (w308:i32)
        n134 = local read "lower threshold"() -> (w319:i32)
        n135 = case shown="True" "cam_dark?" {
          tunnel: w328 -> [_ w350]
          tunnel: [w347 w349] -> w320
          tunnel: w321 -> [w347 w348]
          frame False {
          }
          frame True {
            n136 = Subtract(x=w348, y=w350) -> (x-y=w349:dbl[][])
          }
        }
        n137 = call "filtr.vi"("lower threshold"=w319, "upper threshold"=w308, "input array"=w320) -> ("output array"=w317:dbl[][])  [unwired: 8 in]
        n138 = call <vilib>:"High Resolution Relative Seconds.vi"() -> ("relative seconds"=w333:dbl)
        n139 = Subtract(x=w333, y=w332) -> (x-y=w331:dbl)
        n140 = Reciprocal(x=w331) -> (1/x=→"cam_fps":dbl)
        n141 = case shown="True" "cam_liveavg" {
          tunnel: w317 -> [w336 w342]
          tunnel: [w336 w338] -> w309
          tunnel: w316 -> [_ w344]
          tunnel: w315 -> [w337 w346]
          tunnel: [w337 w345] -> w314
          tunnel: w313 -> [_ w345]
          frame False {
          }
          frame True {
            n142 = Subtract(x=w346, y=w345) -> (x-y=w340:i32)
            n143 = Multiply(x=w344, y=w340) -> (x*y=w343:dbl[][])
            n144 = Increment(x=w340) -> (x+1=w339:i32)
            n145 = Add(x=w343, y=w342) -> (x+y=w341:dbl[][])
            n146 = Divide(x=w341, y=w339) -> (x/y=w338:dbl[][])
          }
        }
        "mainimg" <- w309
        n147 = Array Max & Min(array=w309) -> (max value=→"max":dbl)  [unwired: 3 out]
        n148 = Add Array Elements(numeric array=w309) -> (sum=→"sum":dbl)
        n149 = Transpose 2D Array(2D array=w309) -> (transposed array=w310:dbl[][])
        n150 = for {
          tunnel: w310 -> [w335] mode=indexing
          tunnel: [w334] -> w311 mode=indexing
          n151 = Add Array Elements(numeric array=w335) -> (sum=w334:dbl)
        }
        "G2" <- w311
      }
      frame "dark" {
        n152 = Dequeue Element(queue=w364) -> ()  [unwired: 2 in, 4 out]
        n153 = Array Size(array=w361) -> (size(s)=w360:i32[])
        n154 = Index Array(array=w360) -> (element #1=w359:i32, element #2=w358:i32)  [unwired: 2 in]
        n155 = Initialize Array(0.0 ("element"), w359, w358) -> (w356:dbl[][])
        n156 = for {
          N: "dark avg" -> [_]
          tunnel: w366 -> [w374]
          tunnel: w365 -> [w373]
          tunnel: [w372] -> w363
          tunnel: w361 -> [w371]
          tunnel: [w370] -> w362
          shift-right: [w367] -> w354
          shift-left: w356 -> [w368]
          n157 = call "grabimg.vi"("array in"=w371, "error in"=w373, "Hin"=w374) -> ("error out"=w372:errorcluster, "imgdata"=w369:i32[][], "Hout"=w370:u64)  [unwired: 6 in]
          n158 = Add(x=w369, y=w368) -> (x+y=w367:dbl[][])
        }
        n159 = Divide(x=w354, y="dark avg") -> (x/y=w355:dbl[][])
      }
      frame "snap" {
        n160 = Dequeue Element(queue=w392) -> ()  [unwired: 2 in, 4 out]
        n161 = local read "cam_dark?"() -> (w391:bool)
        n162 = local read "averages"() -> (w386:i32)
        n163 = To Double Precision Float(number=w381) -> (double precision float=w380:dbl[][])
        n164 = Equal To 0?(x="aq.mode") -> (x = 0?=w377:bool)
        n165 = Get Date/Time In Seconds() -> (seconds since 1Jan1904=w382:timestamp)
        n166 = for {
          N: w386 -> [w409]
          shift-right: [w420] -> w387
          shift-left: w389 -> [w422]
          shift-right: [w403] -> w385
          shift-left: w388 -> [w421]
          tunnel: w391 -> [w418]
          tunnel: w390 -> [w417]
          tunnel: w381 -> [w416]
          tunnel: w382 -> [w411]
          tunnel: w377 -> [w394]
          shift-right: [w393] -> w376
          shift-left: w380 -> [w396]
          i -> [w395]
          n167 = call "grabimg.vi"("array in"=w416, "error in"=w421, "Hin"=w422) -> ("error out"=w403:errorcluster, "imgdata"=w419:i32[][], "Hout"=w420:u64)  [unwired: 6 in]
          n168 = local read "upper threshold"() -> (w402:i32)
          n169 = local read "lower threshold"() -> (w398:i32)
          n170 = case shown="True" w418 {
            tunnel: w419 -> [w444 w447]
            tunnel: w417 -> [_ w446]
            tunnel: [w444 w445] -> w415
            frame False {
            }
            frame True {
              n171 = Subtract(x=w447, y=w446) -> (x-y=w445:dbl[][])
            }
          }
          n172 = Get Date/Time In Seconds() -> (seconds since 1Jan1904=w414:timestamp)
          n173 = Subtract(x=w414, y=w411) -> (x-y=w413:dbl)
          n174 = call "filtr.vi"("lower threshold"=w398, "upper threshold"=w402, "input array"=w415) -> ("output array"=w401:dbl[][])  [unwired: 8 in]
          n175 = Divide(x=w413, y=w395) -> (x/y=w407:dbl)
          n176 = Reciprocal(x=w407) -> (1/x=w406:dbl)
          n177 = Multiply(x=w407, y=w409) -> (x*y=w412:dbl)
          n178 = Divide(x=w409, y=w395) -> (x/y=→"snap_prog":dbl)
          n179 = case shown="False" "count?" {
            tunnel: w401 -> [w433 w435]
            tunnel: "e-size" -> [_ w437]
            tunnel: w398 -> [_ w436]
            tunnel: [w433 w434] -> w397
            frame False {
            }
            frame True {
              n180 = Array Size(array=w435) -> (size(s)=w439:i32[])
              n181 = call "findr.vi"("thresh"=w436, "esize"=w437, "inp array"=w435) -> ("locs"=w438:i32[][])  [unwired: 8 in]
              n182 = Index Array(array=w439) -> (element #1=w441:i32, element #2=w440:i32)  [unwired: 2 in]
              n183 = call "drawe.vi"("Ysize"=w441, "Xsize"=w440, "pos array"=w438) -> ("img out"=w434:i32[][])  [unwired: 8 in]
            }
          }
          n184 = Add(x=w412, y=w411) -> (x+y=→"ETA":timestamp)
          n185 = local write "cam_fps"(w406) -> ()
          n186 = case shown="True" w394 {
            tunnel: w397 -> [w423 w431]
            tunnel: w395 -> [_ w430]
            tunnel: w396 -> [w425 w429]
            tunnel: [w424 w426] -> w393
            frame False {
              n187 = Add(x=w423, y=w425) -> (x+y=w424:dbl[][])
            }
            frame True {
              n188 = Multiply(x=w429, y=w430) -> (x*y=w432:dbl[][])
              n189 = Increment(x=w430) -> (x+1=w427:i32)
              n190 = Add(x=w431, y=w432) -> (x+y=w428:dbl[][])
              n191 = Divide(x=w428, y=w427) -> (x/y=w426:dbl[][])
            }
          }
          n192 = local write "mainimg"(w401) -> ()
          n193 = Transpose 2D Array(2D array=w401) -> (transposed array=w404:dbl[][])
          n194 = for {
            tunnel: w404 -> [w443] mode=indexing
            tunnel: [w442] -> w405 mode=indexing
            n195 = Add Array Elements(numeric array=w443) -> (sum=w442:dbl)
          }
          n196 = local write "sideimg"(w393) -> ()
          n197 = local write "G2"(w405) -> ()
        }
        n198 = Enqueue Element(queue=w379, element=w376, error in (no error)=w385) -> (error out=w375:errorcluster)  [unwired: 1 in, 2 out]
      }
      frame "suspend" {
        n199 = Dequeue Element(queue=w455) -> ()  [unwired: 2 in, 4 out]
      }
    }
    "cam_error" <- w218
  }
  n200 = while {
    tunnel: w9 -> [w461]
    tunnel: w12 -> [w460]
    tunnel: w24 -> [w459]
    tunnel: w23 -> [w458]
    tunnel: w1 -> [w456]
    tunnel: w10 -> [w457]
    stop <- w462 stop-if-true
    n201 = event shown="[10] \"cam_saveimg\": Value Change" {
      selector: _ -> [_ _ _ _ _ _ _ _ _ _ _ _ _ _ _ _ _ _ _ _]
      dyn-events: _ -> [_ _ _ _ _ _ _ _ _ _ _ _ _ _ _ _ _ _ _ _]
      timeout: _ -> [_ _ _ _ _ _ _ _ _ _ _ _ _ _ _ _ _ _ _ _]
      tunnel: [_ TRUE _ _ _ _ _ _ _ _ _ _ _ _ _ _ _ _ _ _] -> w462
      tunnel: w461 -> [_ w474 w477 _ _ _ _ _ w503 w505 _ _ _ _ _ _ _ _ _ _]
      tunnel: w460 -> [_ w473 _ w481 _ _ _ _ _ _ _ _ _ _ _ w517 _ w529 _ _]
      tunnel: w459 -> [_ w472 _ _ w487 _ _ _ _ _ _ _ _ _ _ _ _ _ _ _]
      tunnel: w458 -> [_ w471 _ _ _ w493 w499 w500 _ _ _ _ _ _ _ _ _ _ _ _]
      tunnel: w457 -> [_ w465 _ _ _ _ _ _ _ _ _ _ _ _ _ _ _ _ _ _]
      tunnel: w456 -> [_ w464 _ _ _ _ _ _ _ _ w507 w509 _ _ _ _ _ _ _ _]
      event Timeout {
        n202 = event-data() -> ()  [unwired: 1 in, 1 out]
      }
      event "main_close": Value Change {
        w463 = "close" ("element")
        w470 = "release" ("element")
        n203 = event-data() -> ()  [unwired: 1 in, 1 out]
        n204 = Release Queue(queue=w465) -> ()  [unwired: 2 in, 3 out]
        n205 = Enqueue Element(queue=w474, element=w470) -> (queue out=w469:refnum<queue>)  [unwired: 2 in, 2 out]
        n206 = Enqueue Element(queue=w473, element=w470) -> (queue out=w468:refnum<queue>)  [unwired: 2 in, 2 out]
        n207 = Enqueue Element(queue=w472, element=w470) -> (queue out=w467:refnum<queue>)  [unwired: 2 in, 2 out]
        n208 = Enqueue Element(queue=w471, element=w470) -> (queue out=w466:refnum<queue>)  [unwired: 2 in, 2 out]
        n209 = Enqueue Element(queue=w469, element=w463) -> ()  [unwired: 2 in, 3 out]
        n210 = Enqueue Element(queue=w468, element=w463) -> ()  [unwired: 2 in, 3 out]
        n211 = Enqueue Element(queue=w467, element=w463) -> ()  [unwired: 2 in, 3 out]
        n212 = Enqueue Element(queue=w466, element=w463) -> ()  [unwired: 2 in, 3 out]
        n213 = Enqueue Element(queue=w464, element=w463) -> ()  [unwired: 2 in, 3 out]
      }
      event "cam_release", "cam_init": Value Change {
        n214 = event-data() -> ()  [unwired: 1 in, 2 out]
        n215 = Select(t="init" ("name (unnamed)"), s="cam_init", f="release" ("name (unnamed)")) -> (s? t:f=w476:string)
        n216 = Enqueue Element(queue=w477, element=w476) -> ()  [unwired: 2 in, 3 out]
      }
      event "ESP_release", "ESP_init": Value Change {
        n217 = event-data() -> ()  [unwired: 1 in, 2 out]
        n218 = Select(t="init" ("name (unnamed)"), s="ESP_init", f="release" ("name (unnamed)")) -> (s? t:f=w485:string)
        n219 = Enqueue Element(queue=w481, element=w485) -> ()  [unwired: 2 in, 3 out]
      }
      event "manip_init", "manip_release": Value Change {
        n220 = event-data() -> ()  [unwired: 1 in, 2 out]
        n221 = Flush Queue(queue=w487) -> (queue out=w486:refnum<queue>)  [unwired: 1 in, 2 out]
        n222 = Select(t="init" ("name (unnamed)"), s="manip_init", f="release" ("name (unnamed)")) -> (s? t:f=w489:string)
        n223 = Enqueue Element(queue=w486, element=w489) -> ()  [unwired: 2 in, 3 out]
      }
      event "phoib_release", "phoib_init": Value Change {
        n224 = event-data() -> ()  [unwired: 1 in, 2 out]
        n225 = Flush Queue(queue=w493) -> (queue out=w492:refnum<queue>)  [unwired: 1 in, 2 out]
        n226 = Select(t="init" ("name (unnamed)"), s="phoib_init", f="release" ("name (unnamed)")) -> (s? t:f=w495:string)
        n227 = Enqueue Element(queue=w492, element=w495) -> ()  [unwired: 2 in, 3 out]
      }
      event "phoib_standby": Value Change {
        n228 = event-data() -> ()  [unwired: 1 in, 2 out]
        n229 = Enqueue Element(queue=w499, element="standby") -> ()  [unwired: 2 in, 3 out]
      }
      event "phoib_set": Value Change {
        n230 = event-data() -> ()  [unwired: 1 in, 2 out]
        n231 = Enqueue Element(queue=w500, element="set") -> ()  [unwired: 2 in, 3 out]
      }
      event "cam_dark": Value Change {
        n232 = event-data() -> ()  [unwired: 1 in, 2 out]
        n233 = Enqueue Element(queue=w503, element="dark") -> ()  [unwired: 2 in, 3 out]
      }
      event "ROI Left", "ROI Right", "ROI Top", "ROI Bottom", "exposure [ms]", "binning", "gain": Value Change {
        n234 = event-data() -> ()  [unwired: 1 in, 1 out]
        n235 = Enqueue Element(queue=w505, element="set") -> ()  [unwired: 2 in, 3 out]
      }
      event "cam_saveimg": Value Change {
        n236 = event-data() -> ()  [unwired: 1 in, 1 out]
        n237 = Enqueue Element(queue=w507, element="single") -> ()  [unwired: 2 in, 3 out]
      }
      event "delscan_go": Value Change {
        n238 = event-data() -> ()  [unwired: 1 in, 1 out]
        n239 = Enqueue Element(queue=w509, element="GO") -> ()  [unwired: 2 in, 3 out]
      }
      event "Move Abs": Value Change {
        n240 = event-data() -> ()  [unwired: 1 in, 1 out]
      }
      event "ManipRel +", "ManipRel -": Value Change {
        n241 = event-data() -> ()  [unwired: 1 in, 2 out]
      }
      event "stop manip": Value Change {
        n242 = event-data() -> ()  [unwired: 1 in, 1 out]
      }
      event "ESP_go": Value Change {
        w511 = ":" ("string")
        n243 = event-data() -> ()  [unwired: 1 in, 1 out]
        n244 = local read "ESP Axis"() -> (w510:i32)
        n245 = Number To Decimal String(number=w510) -> (decimal integer string=w513:string)  [unwired: 1 in]
        n246 = Number To Fractional String(number="ESP_dest") -> (F-format string=w512:string)  [unwired: 3 in]
        n247 = Concatenate Strings("abs:" ("string"), w513, w511, w512, w511) -> (w516:string)
        n248 = Enqueue Element(queue=w517, element=w516) -> ()  [unwired: 2 in, 3 out]
      }
      event "ESP_set_t0": Value Change {
        n249 = event-data() -> ()  [unwired: 1 in, 1 out]
        n250 = Current VI's Path() -> (path=w523:path)
        n251 = Strip Path(path=w523) -> (stripped path=w519:path)  [unwired: 1 out]
        n252 = Strip Path(path=w519) -> (stripped path=w518:path)  [unwired: 1 out]
        n253 = local read "ESP_pos"() -> (w521:dbl)
        "ESP_t0" <- w521
        n254 = Number To Fractional String(number=w521) -> (F-format string=w520:string)  [unwired: 3 in]
        n255 = Build Path(base path=w518, name or relative path="t0.txt") -> (appended path=w522:path)
        n256 = Write to Text File(file (use dialog)=w522, text=w520) -> ()  [unwired: 2 in, 3 out]
      }
      event "ESP_+", "ESP_-": Value Change {
        n257 = event-data() -> ()  [unwired: 1 in, 6 out]
        n258 = Negate(x="ESP_delta") -> (-x=w532:dbl)
        n259 = Select(t="ESP_delta", s="ESP_+", f=w532) -> (s? t:f=w530:dbl)
        n260 = Number To Decimal String(number="ESP Axis") -> (decimal integer string=w527:string)  [unwired: 1 in]
        n261 = Number To Fractional String(number=w530) -> (F-format string=w525:string)  [unwired: 3 in]
        n262 = Concatenate Strings("rel:" ("string"), w527, ":" ("string"), w525) -> (w535:string)
        n263 = Enqueue Element(queue=w529, element=w535) -> ()  [unwired: 2 in, 3 out]
      }
      event "ESP_dest": Value Change {
        n264 = event-data() -> ()  [unwired: 1 in, 6 out]
        n265 = local read "ESP_dest"() -> (w539:dbl)
        n266 = local read "ESP_t0"() -> (w538:dbl)
        n267 = call "mm2time.vi"("fs?"=TRUE ("fs[1]/ps[0]"), "Offset (mm)"=w538, "distance (mm)"=w539) -> ("time in fs/ps seconds"=w536:dbl)
        n268 = local write "ESP_dest_t"(w536) -> ()
      }
      event "ESP_dest_t": Value Change {
        n269 = event-data() -> ()  [unwired: 1 in, 1 out]
        n270 = local read "ESP_t0"() -> (w542:dbl)
        n271 = call "time2mm.vi"("fs[1]/ps[0]"=TRUE, "Offset (mm)"=w542, "time"="ESP_dest_t") -> ("position (mm)"=w540:dbl)
        n272 = local write "ESP_dest"(w540) -> ()
      }
    }
  }
  n273 = while {
    tunnel: w12 -> [w552]
    shift-right: [w550] -> _
    shift-left: _ -> [w548]
    shift-right: [w549] -> _
    shift-left: _ -> [w547]
    shift-right: [w545] -> _
    shift-left: 0 -> [w546]
    tunnel: w1 -> [w544]
    stop <- w551 stop-if-true
    # "ESP"
    n274 = Preview Queue Element(queue=w552, timeout in ms (-1)=w546) -> (queue out=w555:refnum<queue>, element=w556:string)  [unwired: 1 in, 2 out]
    n275 = Match Pattern(string=w556, regular expression=":") -> (before substring=w554:string, after substring=w553:string)  [unwired: 1 in, 2 out]
    n276 = case shown="\"abs\"" w554 {
      tunnel: w555 -> [_ w567 w585 w619 w620 w627 w632]
      tunnel: w553 -> [_ w572 w592 _ _ _ _]
      tunnel: [_ _ _ _ _ TRUE _] -> w551
      tunnel: [w559 w574 w586 w617 refnum<visa-resource-name> refnum ("VISA resource name out") w624 w631] -> w550
      tunnel: [w558 w575 w584 w616 w622 w625 w630] -> w549
      tunnel: w548 -> [w563 w577 w590 w617 w623 w624 _]
      tunnel: w547 -> [w562 w576 w591 w616 _ w625 _]
      tunnel: [_ _ _ -1 _ _ _] -> w545
      tunnel: w544 -> [_ _ w583 _ _ _ _]
      frame "idle", Default {
        n277 = local read "ESP Axis"() -> (w560:i32)
        n278 = local read "ESP_t0"() -> (w566:dbl)
        n279 = call "Read Actual Position.vi"("error in (no error)"=w562, "Axis (1)"=w560, "VISA resource name"=w563) -> ("error out"=w558:errorcluster, "Position (units)"=w561:dbl, "VISA resource name out"=w559:refnum<visa-resource-name>)  [unwired: 2 in]
        "ESP_pos" <- w561
        n280 = call "mm2time.vi"("fs?"=TRUE, "Offset (mm)"=w566, "distance (mm)"=w561) -> ("time in fs/ps seconds"=→"ESP_delay":dbl)
      }
      frame "rel" {
        n281 = Match Pattern(string=w572, regular expression=":") -> (before substring=w571:string, after substring=w570:string)  [unwired: 1 in, 2 out]
        n282 = Dequeue Element(queue=w567) -> ()  [unwired: 2 in, 4 out]
        n283 = Decimal String To Number(string=w571) -> (number=w569:i32)  [unwired: 2 in, 1 out]
        n284 = Fract/Exp String To Number(string=w570) -> (number=w568:dbl)  [unwired: 3 in, 1 out]
        n285 = call "Move Relative.vi"("error in (no error)"=w576, "Position (0 units)"=w568, "Axis (1)"=w569, "VISA resource name"=w577) -> ("error out"=w575:errorcluster, "VISA resource name out"=w574:refnum<visa-resource-name>)  [unwired: 2 in]
      }
      frame "abs" {
        n286 = Dequeue Element(queue=w585) -> ()  [unwired: 2 in, 4 out]
        n287 = Match Pattern(string=w592, regular expression=":") -> (before substring=w593:string, after substring=w581:string)  [unwired: 1 in, 2 out]
        n288 = Match Pattern(string=w581, regular expression=":") -> (before substring=w580:string, after substring=w579:string)  [unwired: 1 in, 2 out]
        n289 = Decimal String To Number(string=w593) -> (number=w589:i32)  [unwired: 2 in, 1 out]
        n290 = Fract/Exp String To Number(string=w580) -> (number=w578:dbl)  [unwired: 3 in, 1 out]
        n291 = call "Move Absolute.vi"("error in (no error)"=w591, "Position (0 units)"=w578, "Axis (1)"=w589, "VISA resource name"=w590) -> ("error out"=w587:errorcluster, "VISA resource name out"=w588:refnum<visa-resource-name>)  [unwired: 2 in]
        n292 = case shown="\"wait\"" w579 {
          tunnel: w589 -> [_ w601]
          tunnel: w588 -> [w596 w606]
          tunnel: w587 -> [w595 w605]
          tunnel: [w596 w598] -> w586
          tunnel: [w595 w604] -> w584
          tunnel: w583 -> [_ w603]
          frame "", Default {
          }
          frame "wait" {
            n293 = while {
              tunnel: w601 -> [w615]
              shift-right: [w612] -> w600
              shift-left: w606 -> [w614]
              shift-right: [w611] -> w599
              shift-left: w605 -> [w613]
              stop <- w610 stop-if-true
              n294 = call "Get Axis Motion Status.vi"("error in (no error)"=w613, "Axis (1)"=w615, "VISA resource name"=w614) -> ("error out"=w611:errorcluster, "Motion Done"=w610:bool, "VISA resource name out"=w612:refnum<visa-resource-name>)  [unwired: 2 in]
            }
            n295 = flat-sequence {
              tunnel: w600 -> [w609]
              tunnel: w599 -> [w608]
              tunnel: [w609] -> w598
              tunnel: [w608] -> w597
              frame #0 {
                n296 = Wait (ms)(milliseconds to wait=u32 1000) -> ()  [unwired: 1 out]
              }
            }
            n297 = Enqueue Element(queue=w603, element="done", error in (no error)=w597) -> (error out=w604:errorcluster)  [unwired: 1 in, 2 out]
          }
        }
      }
      frame "suspend" {
        n298 = Dequeue Element(queue=w619) -> ()  [unwired: 2 in, 4 out]
      }
      frame "release" {
        n299 = Dequeue Element(queue=w620) -> ()  [unwired: 2 in, 4 out]
        n300 = call "Close.vi"("VISA resource name"=w623) -> ("error out"=w622:errorcluster)  [unwired: 10 in]
      }
      frame "close" {
        n301 = Release Queue(queue=w627) -> ()  [unwired: 2 in, 3 out]
      }
      frame "init" {
        n302 = Dequeue Element(queue=w632) -> ()  [unwired: 2 in, 4 out]
        n303 = flat-sequence {
          tunnel: [w635] -> w629
          tunnel: [w634] -> w628
          tunnel: [w639] -> w630
          tunnel: [w640] -> w631
          tunnel: w629 -> [w640]
          tunnel: w628 -> [w639]
          frame #0 {
            n304 = local write "ESP_con?"(FALSE ("ESP_con?")) -> ()
          }
          frame #1 {
            n305 = call "Initialize.vi"("VISA resource name"="ESP301 VISA", "Serial Link (RS232)"=enum16{"RS232", "USB"}."USB") -> ("VISA resource name out"=w635:refnum<visa-resource-name>, "error out"=w634:errorcluster)  [unwired: 7 in]
          }
          frame #2 {
            n306 = local write "ESP_con?"(TRUE ("ESP_con?")) -> ()
          }
        }
      }
    }
  }
  n307 = while {
    tunnel: w24 -> [w648]
    shift-right: [w646] -> _
    shift-left: _ -> [w644]
    shift-right: [w645] -> _
    shift-left: _ -> [w643]
    shift-right: [w641] -> _
    shift-left: 0 -> [w642]
    stop <- w647 stop-if-true
    # "manip"
    n308 = Preview Queue Element(queue=w648, timeout in ms (-1)=w642) -> (queue out=w651:refnum<queue>, element=w652:string)  [unwired: 1 in, 2 out]
    n309 = Match Pattern(string=w652, regular expression=":") -> (before substring=w650:string, after substring=w649:string)  [unwired: 1 in, 2 out]
    n310 = case shown="\"relative\"" w650 {
      tunnel: w651 -> [_ w669 w679 w683 w692 w703]
      tunnel: w649 -> [_ w671 _ _ _ _]
      tunnel: [_ _ _ _ TRUE _] -> w647
      tunnel: [w655 w657 w681 refnum<k5> refnum ("gateway_connection out") w690 w694] -> w646
      tunnel: [w654 w656 w680 w685 w689 w693] -> w645
      tunnel: w644 -> [w655 w673 w681 w687 w690 _]
      tunnel: w643 -> [w654 w672 w680 _ w689 _]
      tunnel: [_ _ -1 _ _ _] -> w641
      frame "idle", Default {
      }
      frame "relative" {
        n311 = Dequeue Element(queue=w669) -> ()  [unwired: 2 in, 4 out]
        n312 = call "sp_manip_get_axis_status.vi"("error in"=w672, "gateway_connection"=w673) -> ("error out"=w675:errorcluster, "axis_out"=w661:T7, "gateway_connection out"=w674:refnum<k5>)  [unwired: 5 in, 2 out]
        n313 = Scan From String(format string="%f_%f_%f_%f_%f_%f", input string=w671) -> (output 1=w668:dbl, output 2=w667:dbl, output 3=w666:dbl, output 4=w665:dbl, output 5=w664:dbl, output 6=w663:dbl)  [unwired: 8 in, 3 out]
        n314 = for {
          tunnel: w661 -> [w678] mode=indexing
          tunnel: [w677] -> w659 mode=indexing
          tunnel: [w676] -> w660 mode=indexing
          n315 = Unbundle By Name(w678) -> ("Axis_Name"=w677:string, "Axis_Position"=w676:dbl)
        }
        n316 = Build Array(w668, w667, w666, w665, w664, w663) -> (w662:dbl[])
        n317 = Add(x=w660, y=w662) -> (x+y=w658:dbl[])
        n318 = call "sp_manip_start_move.vi"("error in"=w675, "target positions"=w658, "axis names"=w659, "gateway_connection"=w674) -> ("error out"=w656:errorcluster, "gateway_connection out"=w657:refnum<k5>)  [unwired: 4 in, 2 out]
      }
      frame "suspend" {
        n319 = Dequeue Element(queue=w679) -> ()  [unwired: 2 in, 4 out]
      }
      frame "release" {
        n320 = Dequeue Element(queue=w683) -> ()  [unwired: 2 in, 4 out]
        n321 = call "sp_manip_disconnect.vi"("gateway_connection"=w687) -> ("error out"=w686:errorcluster, "gateway_connection_out"=w688:refnum<k5>)  [unwired: 7 in, 2 out]
        n322 = call "tcp_gateway_close_connection.vi"("error in"=w686, "server_connection"=w688) -> ("error out"=w685:errorcluster)  [unwired: 5 in]
      }
      frame "close" {
        n323 = Release Queue(queue=w692) -> ()  [unwired: 2 in, 3 out]
      }
      frame "init" {
        n324 = Dequeue Element(queue=w703) -> ()  [unwired: 2 in, 4 out]
        n325 = call "tcp_gateway_open_connection.vi"() -> ("gateway_connection"=w698:refnum<k5>, "error out"=w697:errorcluster)  [unwired: 5 in, 3 out]
        n326 = call "sp_manip_connect.vi"("error in"=w697, "gateway_connection"=w698) -> ("error out"=w693:errorcluster, "axis_out"=w696:T7, "gateway_connection out"=w694:refnum<k5>)  [unwired: 5 in, 2 out]
        n327 = for {
          tunnel: w696 -> [w706] mode=indexing
          tunnel: [w705] -> w701 mode=indexing
          tunnel: [w704] -> w702 mode=indexing
          n328 = Unbundle By Name(w706) -> ("Axis_Name"=w705:string, "Axis_Position"=w704:dbl)
        }
        "axis" <- w701
        "pos" <- w702
        n329 = control-ref of="meas_axis"() -> (w695:refnum<vi>)
        n330 = local write "dest"(w702) -> ()
        n331 = Build Array (concatenate)(w701, "XY") -> (w699:string[])
        n332 = property on="Property Node" class="CmbBox"(reference=w695, "Strings[]"=w699) -> ()  [unwired: 1 in, 2 out]
      }
    }
  }
  n333 = while {
    tunnel: w23 -> [w717]
    shift-right: [w714] -> _
    shift-left: 0 -> [w715]
    shift-right: [w713] -> _
    shift-left: _ -> [w712]
    shift-right: [w711] -> _
    shift-left: _ -> [w710]
    shift-right: [w709] -> _
    shift-left: u32 0 ("pHandle") -> [w708]
    tunnel: string[] ["Kinetic Energy", "Pass Energy", "Coil Current", "Work Function", "Detector Voltage", "Screen Voltage", "Conversion Voltage", "Focus Displacement 1", "Focus Displacement 2"] -> [w707]
    stop <- w716 stop-if-true
    # "phoib"
    n334 = Preview Queue Element(queue=w717, timeout in ms (-1)=w715) -> (queue out=w720:refnum<queue>, element=w721:string)  [unwired: 1 in, 2 out]
    n335 = Match Pattern(string=w721, regular expression=":") -> (before substring=w719:string, after substring=w718:string)  [unwired: 1 in, 2 out]
    n336 = case shown="\"set\"" w719 {
      tunnel: w720 -> [_ w774 w790 w806 w820 w824 w830]
      tunnel: w718 -> [_ _ _ _ _ _ _]
      tunnel: [_ _ _ _ TRUE _ _] -> w716
      tunnel: [_ _ _ _ _ -1 _] -> w714
      tunnel: [w731 w776 w793 w804 w818 w823 w827] -> w713
      tunnel: w712 -> [w742 w765 w795 w805 w818 w823 _]
      tunnel: [w730 w775 w792 w803 w816 w821 w826] -> w711
      tunnel: w710 -> [w740 w764 w794 _ w816 w821 _]
      tunnel: [w728 w762 w791 w802 w817 w822 w829] -> w709
      tunnel: w708 -> [w728 w762 w791 w801 w817 w822 _]
      tunnel: w707 -> [w729 w755 _ _ _ _ _]
      frame "idle", Default {
        n337 = call "SL2_AD_DLL_Phoibos_GetDeviceState.vi"("dll_path"=w742, "pHandle_in"=w728, "dev_type"=DEF_dev_type."devA (analyzer)", "error in"=w740) -> ("path out"=w727:path, "state"=→"state":T3, "error out"=w726:errorcluster)  [unwired: 2 in]
        n338 = for {
          tunnel: w728 -> [w749]
          tunnel: w729 -> [w747] mode=indexing
          tunnel: [w746] -> w739 mode=indexing
          tunnel: [w745] -> w731
          shift-right: [w744] -> w730
          shift-left: w726 -> [w748]
          tunnel: w727 -> [w743]
          n339 = call "SL2_AD_DLL_Phoibos_GetVoltage.vi"("error in"=w748, "voltage_name"=w747, "pHandle"=w749, "dll path in"=w743) -> ("error out"=w744:errorcluster, "value"=w746:dbl, "dll path out"=w745:path)  [unwired: 3 in]
        }
        n340 = Index Array(array=w739) -> (element #1=→"phoib_I_1":dbl, element #2=→"phoib_I_2":dbl, element #3=→"phoib_I_3":dbl, element #4=→"phoib_I_4":dbl, element #5=→"phoib_I_5":dbl, element #6=→"phoib_I_6":dbl, element #7=→"phoib_I_7":dbl, element #8=→"phoib_I_8":dbl, element #9=→"phoib_I_9":dbl)  [unwired: 9 in]
      }
      frame "set" {
        n341 = Dequeue Element(queue=w774) -> ()  [unwired: 2 in, 4 out]
        n342 = Multiply(x="VoltageRange", y=13) -> (x*y=w771:i32)
        n343 = Add(x="Mode", y=w771) -> (x+y=w768:i32)
        n344 = Index Array(array=u32[] [251749632, 251749633, 251749634, 251749635, 251749636, 251749637, 251749638, 251749639, 251749640, 251749641, 251749642, 251749643, 251749644, 251749645, 251749646, 251749647, 251749648, 251749649, 251749650, 251749651, 251749652, 251749653, 251749654, 251749655, 251749656, 251749657, 251749658, 251749659, 251749660, 251749661, 251749662, 251749663, 251749664, 251749665, 251749666, 251749667, 251749668, 251749669, 251749670, 251749671, 251749672, 251749673, 251749674, 251749675, 251749676, 251749677, 251749678, 251749679, 251749680, 251749681, 251749682, 251749683, 251749684, 251749685, 251749686, 251749687, 251749688, 251749689, 251749690, 251749691, 251749692, 251749693, 251749694, 251749695, 251749696] ("modeIDs"), index=w768) -> (element=w766:u32)
        n345 = Build Array("phoib_I_1s", "phoib_I_2s", "phoib_I_3s", "phoib_I_4s", "phoib_I_5s", "phoib_I_6s", "phoib_I_7s", "phoib_I_8s", "phoib_I_9s") -> (w754:dbl[])
        n346 = call "SL2_AD_DLL_Phoibos_SetDeviceMode.vi"("pHandle"=w762, "error in"=w764, "value"=w766, "dev_type"=DEF_dev_type."devA (analyzer)", "dll path in"=w765) -> ("error out"=w753:errorcluster, "dll path out"=w763:path)  [unwired: 4 in]
        n347 = for {
          tunnel: w762 -> [w782]
          shift-right: [w789] -> w776
          shift-left: w763 -> [w786]
          tunnel: w755 -> [w781] mode=indexing
          tunnel: w754 -> [w780] mode=indexing
          shift-right: [w788] -> w775
          shift-left: w753 -> [w784]
          n348 = call "SL2_AD_DLL_Phoibos_GetVoltageRange.vi"("error in"=w784, "voltage_name"=w781, "pHandle"=w782, "dll path in"=w786) -> ("error out"=w783:errorcluster, "min"=w778:dbl, "max"=w779:dbl, "dll path out"=w785:path)  [unwired: 2 in]
          n349 = In Range and Coerce(upper limit=w779, x=w780, lower limit=w778) -> (coerced(x)=w777:dbl)  [unwired: 1 out]
          n350 = call "SL2_AD_DLL_Phoibos_SetVoltage.vi"("commit"=TRUE, "pHandle"=w782, "error in"=w783, "value"=w777, "voltageName"=w781, "dll path in"=w785) -> ("error out"=w788:errorcluster, "dll path out"=w789:path)  [unwired: 3 in]
        }
      }
      frame "standby" {
        w796 = T3 0 items=["Off"=-1, "Standby"=0, "On"=1] ("state")
        n351 = Dequeue Element(queue=w790) -> ()  [unwired: 2 in, 4 out]
        n352 = call "SL2_AD_DLL_Phoibos_SetDeviceState.vi"("pHandle_in"=w791, "error in"=w794, "state"=w796, "dev_type"=DEF_dev_type."devA (analyzer)", "dll_path"=w795) -> ("error out"=w792:errorcluster, "path out"=w793:path)  [unwired: 2 in]
      }
      frame "release" {
        n353 = Dequeue Element(queue=w806) -> ()  [unwired: 2 in, 4 out]
        n354 = flat-sequence {
          tunnel: w805 -> [w807]
          tunnel: w801 -> [w808]
          tunnel: [w811] -> w800
          tunnel: [w810] -> w799
          tunnel: [u32 0] -> w798
          tunnel: [w813] -> w802
          tunnel: [w814] -> w803
          tunnel: [w815] -> w804
          tunnel: w800 -> [w815]
          tunnel: w799 -> [w814]
          tunnel: w798 -> [w813]
          frame #0 {
            n355 = call "SL2_AD_DLL_Phoibos_Shutdown.vi"("pHandle"=w808, "dll path in"=w807) -> ("error out"=w810:errorcluster, "dll path out"=w811:path)  [unwired: 4 in]
          }
          frame #1 {
            n356 = local write "phoib_con?"(FALSE ("phoib_con?")) -> ()
          }
        }
      }
      frame "close" {
        n357 = Release Queue(queue=w820) -> ()  [unwired: 2 in, 3 out]
      }
      frame "suspend" {
        n358 = Dequeue Element(queue=w824) -> ()  [unwired: 2 in, 4 out]
      }
      frame "init" {
        n359 = Dequeue Element(queue=w830) -> ()  [unwired: 2 in, 4 out]
        n360 = flat-sequence {
          tunnel: [w837] -> w828
          tunnel: [w833] -> w827
          tunnel: [w832] -> w826
          tunnel: [w845] -> w829
          tunnel: w828 -> [w845]
          frame #0 {
            n361 = local write "phoib_con?"(FALSE ("phoib_con?")) -> ()
          }
          frame #1 {
            w836 = DEF_dev_type."devA (analyzer)" ("dev_type")
            n362 = call "GetSL2AD_VI_dllPath.vi"() -> ("error"=w840:errorcluster, "Path"=w841:path)  [unwired: 9 in, 1 out]
            n363 = call "SL2_AD_DLL_List_Devices.vi"("error in"=w840, "dev_type"=w836, "dll path in"=w841) -> ("error out"=w834:errorcluster, "devices"=w843:string[], "dll path out"=w835:path)  [unwired: 2 in]
            n364 = Index Array(array=w843) -> (element=w842:string)  [unwired: 1 in]
            n365 = call "SL2_AD_DLL_Phoibos_Initialize.vi"("error in"=w834, "analyzerId"=w842, "dll_path"=w835) -> ("error out"=w838:errorcluster, "pHandle"=w837:u32, "path out"=w839:path)  [unwired: 2 in]
            n366 = call "SL2_AD_DLL_Phoibos_ListDeviceModes.vi"("dll path in"=w839, "dev_type"=w836, "pHandle"=w837, "error in"=w838) -> ("dll path out"=w833:path, "error out"=w832:errorcluster)  [unwired: 1 in, 2 out]
          }
          frame #2 {
            n367 = local write "phoib_con?"(TRUE ("phoib_con?")) -> ()
          }
        }
      }
    }
    "phoib_error" <- w711
  }
